vi "Main.vi"(11 "Module Admin":refnum<class "Delacor_lib_QMH_Module Admin.lvclass">) -> ()   [LabVIEW 2024, in "Anode.lvlib"]
doc: "This template is based from the Queued Message Handler design pattern and the Queued Message Handler Project Template that ships with LabVIEW 2014.\n\nThe main difference is that the Queue is private to this module and communication between modules is done via Broadcast and Request events.\n\nRequest events are wrapped via public API methods and are handled in the Event handler loop in this VI.\nAny module can register for Broadcast events sent by this module.\n\nThe Event Handling Loop generates messages based on user interface actions.\n\nThe Message Handling Loop processes messages generated by the Event Handling Loop, or by other messages. The messages are string values, so new messages can be added easily to the Message Cases case structure in the Message Handling Loop. Each message cluster can also provide an optional value for Message Data, which is a variant that can be converted to whatever message-specific data is required.\n_____\nBased on Delacor QMH Project Template 3.1.0.34.\n\n<b>Note:</b> This VI was modified by the <b>Validate DQMH Module</b> tool to add a call to the Error Reported VI at the end of the 'Exit' MHL frame.\n\n<b>Note:</b> This VI was modified by the <b>Validate DQMH Module</b> tool to call the Release Message Queue VI in the top-level Error case.\n\n<b>Note:</b> This VI was modified by the <b>Validate DQMH Module</b> tool to wrap the FP.Open method in the module close code with a Conditional Disable Structure so it does not execute when the Main VI is running as a built EXE."
uses:
  Anode.lvlib
  <vilib>/Delacor/Delacor QMH/Libraries/Module Admin_class/Delacor_lib_QMH_Module Admin.lvclass
  <vilib>/MGI/Panel Manager/Panel/Panel/Panel.lvclass
  Modbus Flexi-Flow API/Fmeasure (F,P1,P2)--cluster.ctl
  Module Data--cluster.ctl
  <vilib>/Plasmionique/MB Master/MB_Master_TCP/MB_Master_TCP.lvclass
  C:/Program Files/National Instruments/LabVIEW 2025/vi.lib/Plasmionique/MB Master/MB_Master/MB_Master.lvclass
  Anode Solenoid Valve--enum.ctl
  Modbus Config--cluster.ctl
  Purge Strategy--cluster.ctl
  Purge Strategy--enum.ctl
  <vilib>/Utility/miscctls.llb/LVPointTypeDef.ctl
  phlair-busch-can-bus/PumpControls.ctl
  phlair-busch-can-bus/CAN Frame Sessions.ctl
  Initialise Pressure Regulator Interface Argument--cluster.ctl
  <vilib>/Delacor/Delacor QMH/Libraries/Message Queue_class/Delacor_lib_QMH_Message Queue.lvclass/Delacor_lib_QMH_Message Queue.ctl
  Read Pressure Regulator Status Argument--cluster.ctl
  Stop Argument--cluster.ctl
  <vilib>/Delacor/Delacor QMH/Libraries/Module Admin_class/Delacor_lib_QMH_Module Admin.lvclass/Delacor_lib_QMH_Module Admin.ctl
  Set Anode Inlet Pressure SP Argument--cluster.ctl
  Set Pressure Regulator Control Function Argument--cluster.ctl
  Modbus Flexi-Flow API/Control Function Values--enum.ctl
  Set Anode Inlet Flow SP Argument--cluster.ctl
  Set Anode Inlet Valve State Argument--cluster.ctl
  Set Anode Gas Supply Valve Argument--cluster.ctl
  Set Purge Valve Argument--cluster.ctl
  Set Purge Strategy Argument--cluster.ctl
  Wake Purge Helper Loop Argument--cluster.ctl
  Reset Counter Argument--cluster.ctl
  Start H2 Sensor Measurement Argument--cluster.ctl
  Stop H2 Sensor Measurement Argument--cluster.ctl
  Modbus Flexi-Flow API/Valve State--enum.ctl
  <vilib>/DAQmx/write.llb/DAQmx Write (Digital Bool 1Line 1Point).vi
  <vilib>/Delacor/Delacor QMH/Libraries/Message Queue_class/Delacor_lib_QMH_Enqueue Message (Single).vi
  <vilib>/Delacor/Delacor QMH/Libraries/Module Admin_class/Delacor_lib_QMH_Get External Launch.vi
  <vilib>/MGI/Panel Manager/Panel/Panel/Window/Window.lvclass
  C:/Program Files/National Instruments/LabVIEW 2025/vi.lib/MGI/Panel Manager/Panel/Panel/Panel.lvclass
  <vilib>/MGI/Panel Manager/Panel/Panel/Window/Window.vi
  <vilib>/DAQmx/miscellaneous.llb/DAQmx Fill In Error Info.vi
  <vilib>/Utility/error.llb/Error Cluster From Error Code.vi
  <vilib>/ErrorRing/Error Ring.xnode
  <vilib>/Delacor/Delacor QMH/Libraries/Message Queue_class/Delacor_lib_QMH_Message Queue.lvclass
  <vilib>/MGI/Panel Manager/Panel/Panel Helper/Panel Helper.lvclass
  Modbus Flexi-Flow API/Bronkhorst Flexi-Flow ModbusTCP API.lvlib
  <vilib>/MGI/Panel Manager/Panel/Panel.lvlib
  phlair-busch-can-bus/phlair-busch-can-bus.lvlib
  <userlib>/_OpenG.lib/error/error.llb/openg_error.lvlib
  <resource>/objmgr/xnet.rc
panel:
  out "H2 Sensor Data":dbl[](array[numeric]) caption="data" format="%.2f"
  out "Counter In":sgl
  out "Data Cluster":T1={"Status"="Initial Message", "MB_TCP session"=refnum, "Flow Rate SP (Valve Shutoff)"=0.0, "Anode Solenoid Valve"=enum."CLOSED", "Fmeasure (F, P1, P2)"={"Fmeasure (F)"=0.0, "Fmeasure (P1)"=0.0, "Fmeasure (P2)"=0.0}, "Anode Status Map"={}, "Modbus Config"={"IP Address"="localhost", "Port (502)"=502, "Slave ID (255)"=255, "Timeout (10000)"=10000}, "DAQmx Task Gas Supply"="", "DAQmx Task Purge Valve"="V203_Anode_Purge_Valve", "Purge Strategy"={"Strategy"=enum."FORCE OFF", "Purge Interval [s]"=30.0, "Purge Duration [s]"=1.0}}
  out "Value":sgl
  out "P2 Setpoint":sgl
  out "Control Function":u16
  out "Fmeasure (F, P1, P2)":T3
  in  "Panel":refnum<class "Panel.lvclass">
  in  "Simulate MHL Error":bool
  in  "Simulate EHL Error":bool
  out "error out":errorcluster
  out "Status":string="Anode Tester sent Stop Message."
  # "This is a template that creates a DQMH Singleton using the MGI Panel Manager Framwork.\n\nImplement your user interface on this front panel. The Panel Manager Framework will manage showing and hiding the panel in the appropriate spot. \n\nSee the block diagram for more information on how to use this template."
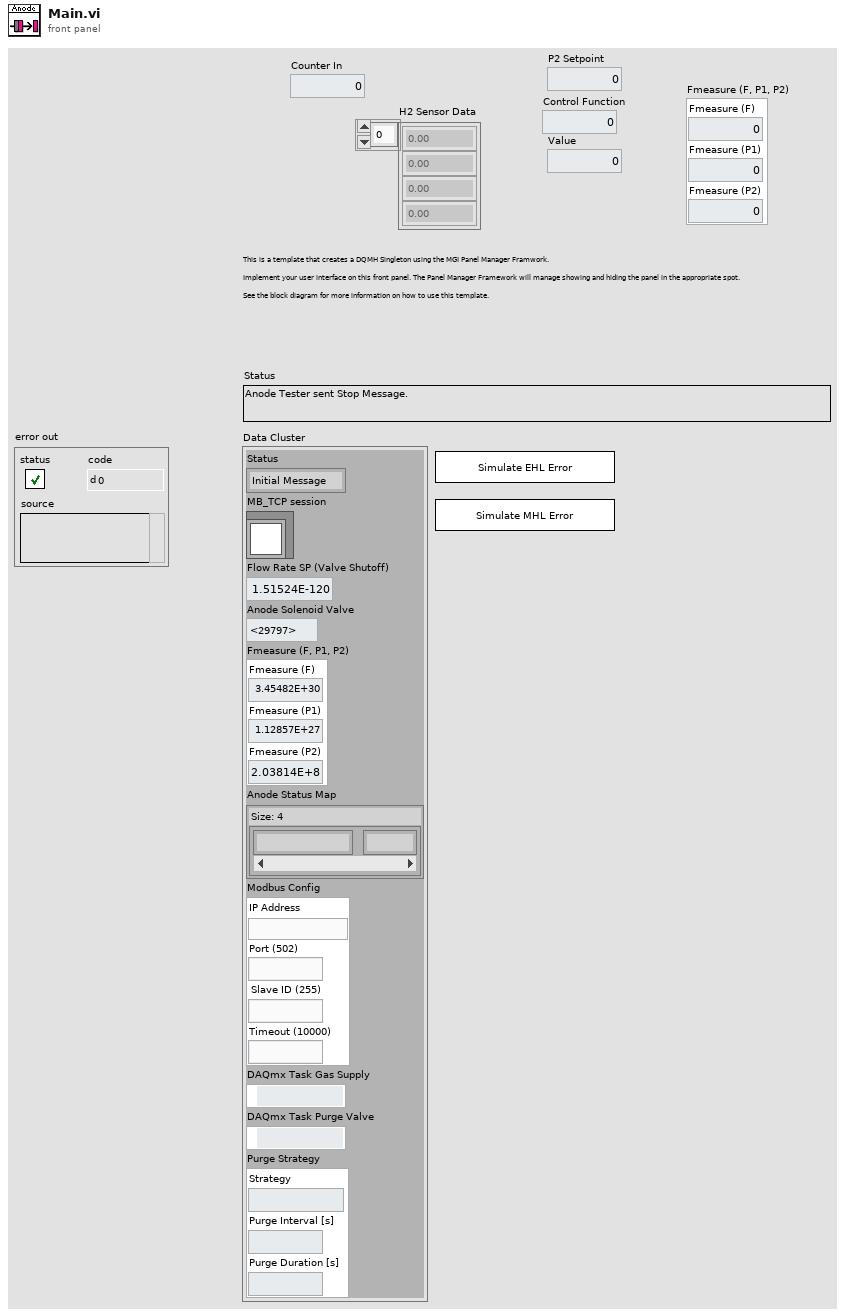
[diagram p1: front panel]
types:
  T1 = typedef "Anode.lvlib/Module Data--cluster.ctl" = cluster{"Status":string, "MB_TCP session":refnum<class "MB_Master_TCP.lvclass">, "Flow Rate SP (Valve Shutoff)":dbl, "Anode Solenoid Valve":T2, "Fmeasure (F, P1, P2)":T3, "Anode Status Map":map{string, dbl}, "Modbus Config":T4, "DAQmx Task Gas Supply":refnum<k21>, "DAQmx Task Purge Valve":refnum<k21>, "Purge Strategy":T5}
  T2 = typedef "Anode.lvlib/Anode Solenoid Valve--enum.ctl" = enum16{"CLOSED", "OPEN"}
  T3 = typedef "Bronkhorst Flexi-Flow ModbusTCP API.lvlib/Fmeasure (F,P1,P2)--cluster.ctl" = cluster{"Fmeasure (F)":sgl, "Fmeasure (P1)":sgl, "Fmeasure (P2)":sgl}
  T4 = typedef "Anode.lvlib/Modbus Config--cluster.ctl" = cluster{"IP Address":string, "Port (502)":u16, "Slave ID (255)":u8, "Timeout (10000)":i32}
  T5 = typedef "Anode.lvlib/Purge Strategy--cluster.ctl" = cluster{"Strategy":T6, "Purge Interval [s]":dbl, "Purge Duration [s]":dbl}
  T6 = typedef "Anode.lvlib/Purge Strategy--enum.ctl" = enum16{"FORCE OFF", "FORCE ON", "TIMED"}
  T7 = typedef "LVPointTypeDef.ctl" = cluster{"Horizontal":i16, "Vertical":i16}
  T8 = typedef "Anode.lvlib/Request Events--cluster.ctl" = cluster{"Stop Module":refnum<user-event>, "Show Panel":refnum<user-event>, "Hide Panel":refnum<user-event>, "Get Module Execution Status":refnum<user-event>, "Show Diagram":refnum<user-event>, "Change Panel":refnum<user-event>, "Set Anode Inlet Pressure SP":refnum<user-event>, "Initialise Pressure Regulator Interface":refnum<user-event>, "Start Polling Pressure Regulator Status":refnum<user-event>, "Stop Polling Pressure Regulator Status":refnum<user-event>, "Read Pressure Regulator Status":refnum<user-event>, "Set Pressure Regulator Control Function":refnum<user-event>, "Set Anode Inlet Flow SP":refnum<user-event>, "Set Anode Inlet Valve State":refnum<user-event>, "Private":cluster{"Wake Connection Helper Loop":refnum<user-event>}, "Set Anode Gas Supply Valve":refnum<user-event>, "Set Purge Valve":refnum<user-event>, "Set Purge Strategy":refnum<user-event>, "Private.Wake Purge Strategy Helper Loop":refnum<user-event>, "Private.Update Purge Strategy Settings":refnum<user-event>, "Wake Purge Helper Loop":refnum<user-event>, "Wake Recirculation Pump Helper Loop":refnum<user-event>, "Sleep Recirculation Pump Helper Loop":refnum<user-event>, "Set Pump Speed SP":refnum<user-event>, "Set Pump Enable State":refnum<user-event>, "Set Pump Speed Control Mode":refnum<user-event>, "Private.Update Purge Strategy Helper Loop":refnum<user-event>, "Force Purge":refnum<user-event>, "Reset Counter":refnum<user-event>, "Private.Wake H2 Sensor Loop":refnum<user-event>, "Private.Sleep H2 Sensor Loop":refnum<user-event>, "Start H2 Sensor Measurement":refnum<user-event>, "Stop H2 Sensor Measurement":refnum<user-event>}
  T9 = typedef "Panel.lvlib/Panel Helper.lvclass/Panel Events.ctl" = cluster{"My Panel":refnum<user-event>, "Top Level Initialized":refnum<user-event>}
  T10 = typedef "phlair-busch-can-bus.lvlib/PumpControls.ctl" = cluster{"Enable Pump":enum16{"DISABLE", "ENABLE"}, "Mass Flow SP [kg/h]":dbl, "Speed SP [U/ min]":u16, "Pump Speed Control":enum16{"DISABLE", "ENABLE"}, "Enable Mass Flow Governer":enum8{"Disable", "Enable", "", "NA"}}
  T11 = typedef "phlair-busch-can-bus.lvlib/CAN Frame Sessions.ctl" = cluster{"Session_Control":refnum<k21>, "Session_Params":refnum<k21>, "Session_Actuals":refnum<k21>, "Session_Acknowledge":refnum<k21>, "Session_H2_Sensor":refnum<k21>}
  T12 = typedef "Anode.lvlib/Initialise Pressure Regulator Interface Argument--cluster.ctl" = cluster{"Modbus Config":T4}
  T13 = typedef "Anode.lvlib/Read Pressure Regulator Status Argument--cluster.ctl" = cluster{"Boolean":bool}
  T14 = typedef "Anode.lvlib/Stop Argument--cluster.ctl" = cluster{"Origin":string, "Exit via Stop Module Req?":bool, "Wait for Module to stop?":bool}
  T15 = typedef "Anode.lvlib/Set Anode Inlet Pressure SP Argument--cluster.ctl" = cluster{"Anode Inlet Pressure [bar]":dbl}
  T16 = typedef "Anode.lvlib/Set Pressure Regulator Control Function Argument--cluster.ctl" = cluster{"Function":T17}
  T17 = typedef "Bronkhorst Flexi-Flow ModbusTCP API.lvlib/Control Function Values--enum.ctl" = enum16{"Flow", "Upstream pressure", "Downstream pressure", "Flow with upstream pressure limit", "Flow with downstream pressure limit", "Upstream pressure with flow limit", "Downstream pressure with flow limit"}
  T18 = typedef "Anode.lvlib/Set Anode Inlet Flow SP Argument--cluster.ctl" = cluster{"Flow SP [slm]":dbl}
  T19 = typedef "Anode.lvlib/Set Anode Inlet Valve State Argument--cluster.ctl" = cluster{"Anode Solenoid Valve":T2}
  T20 = typedef "Anode.lvlib/Set Anode Gas Supply Valve Argument--cluster.ctl" = cluster{"Valve State":enum16{"CLOSED", "OPEN"}}
  T21 = typedef "Anode.lvlib/Set Purge Valve Argument--cluster.ctl" = cluster{"Valve State":enum16{"CLOSED", "OPEN"}}
  T22 = typedef "Anode.lvlib/Set Purge Strategy Argument--cluster.ctl" = cluster{"Purge Controller":T5}
  T23 = typedef "Anode.lvlib/Wake Purge Helper Loop Argument--cluster.ctl" = cluster{"Boolean":bool}
  T24 = typedef "Anode.lvlib/Reset Counter Argument--cluster.ctl" = cluster{"Boolean":bool}
  T25 = typedef "Anode.lvlib/Start H2 Sensor Measurement Argument--cluster.ctl" = cluster{"Boolean":bool}
  T26 = typedef "Anode.lvlib/Stop H2 Sensor Measurement Argument--cluster.ctl" = cluster{"Boolean":bool}
  T27 = enum32{"invalid lock state", "Not Locked", "Locked (No Password)", "Password-protected"}
  T28 = typedef "Bronkhorst Flexi-Flow ModbusTCP API.lvlib/Valve State--enum.ctl" = enum16{"Close", "Open"}
  T29 = enum16{"No reset", "Reset counter", "Reset alarm", "Reset counter (all)", "Reset and disable counter", "Reset firmware program (soft reset)", "Reset Alarm infor error bit", "Reset Alarm info warning bit"}
  T30 = typedef "Anode.lvlib/Purge Valve State--cluster.ctl" = enum16{"WAITING", "PURGING"}
  T31 = cluster{"Timestamp Latest Purge":timestamp, "Timestamp Purge Start":timestamp, "Purge State":T30}
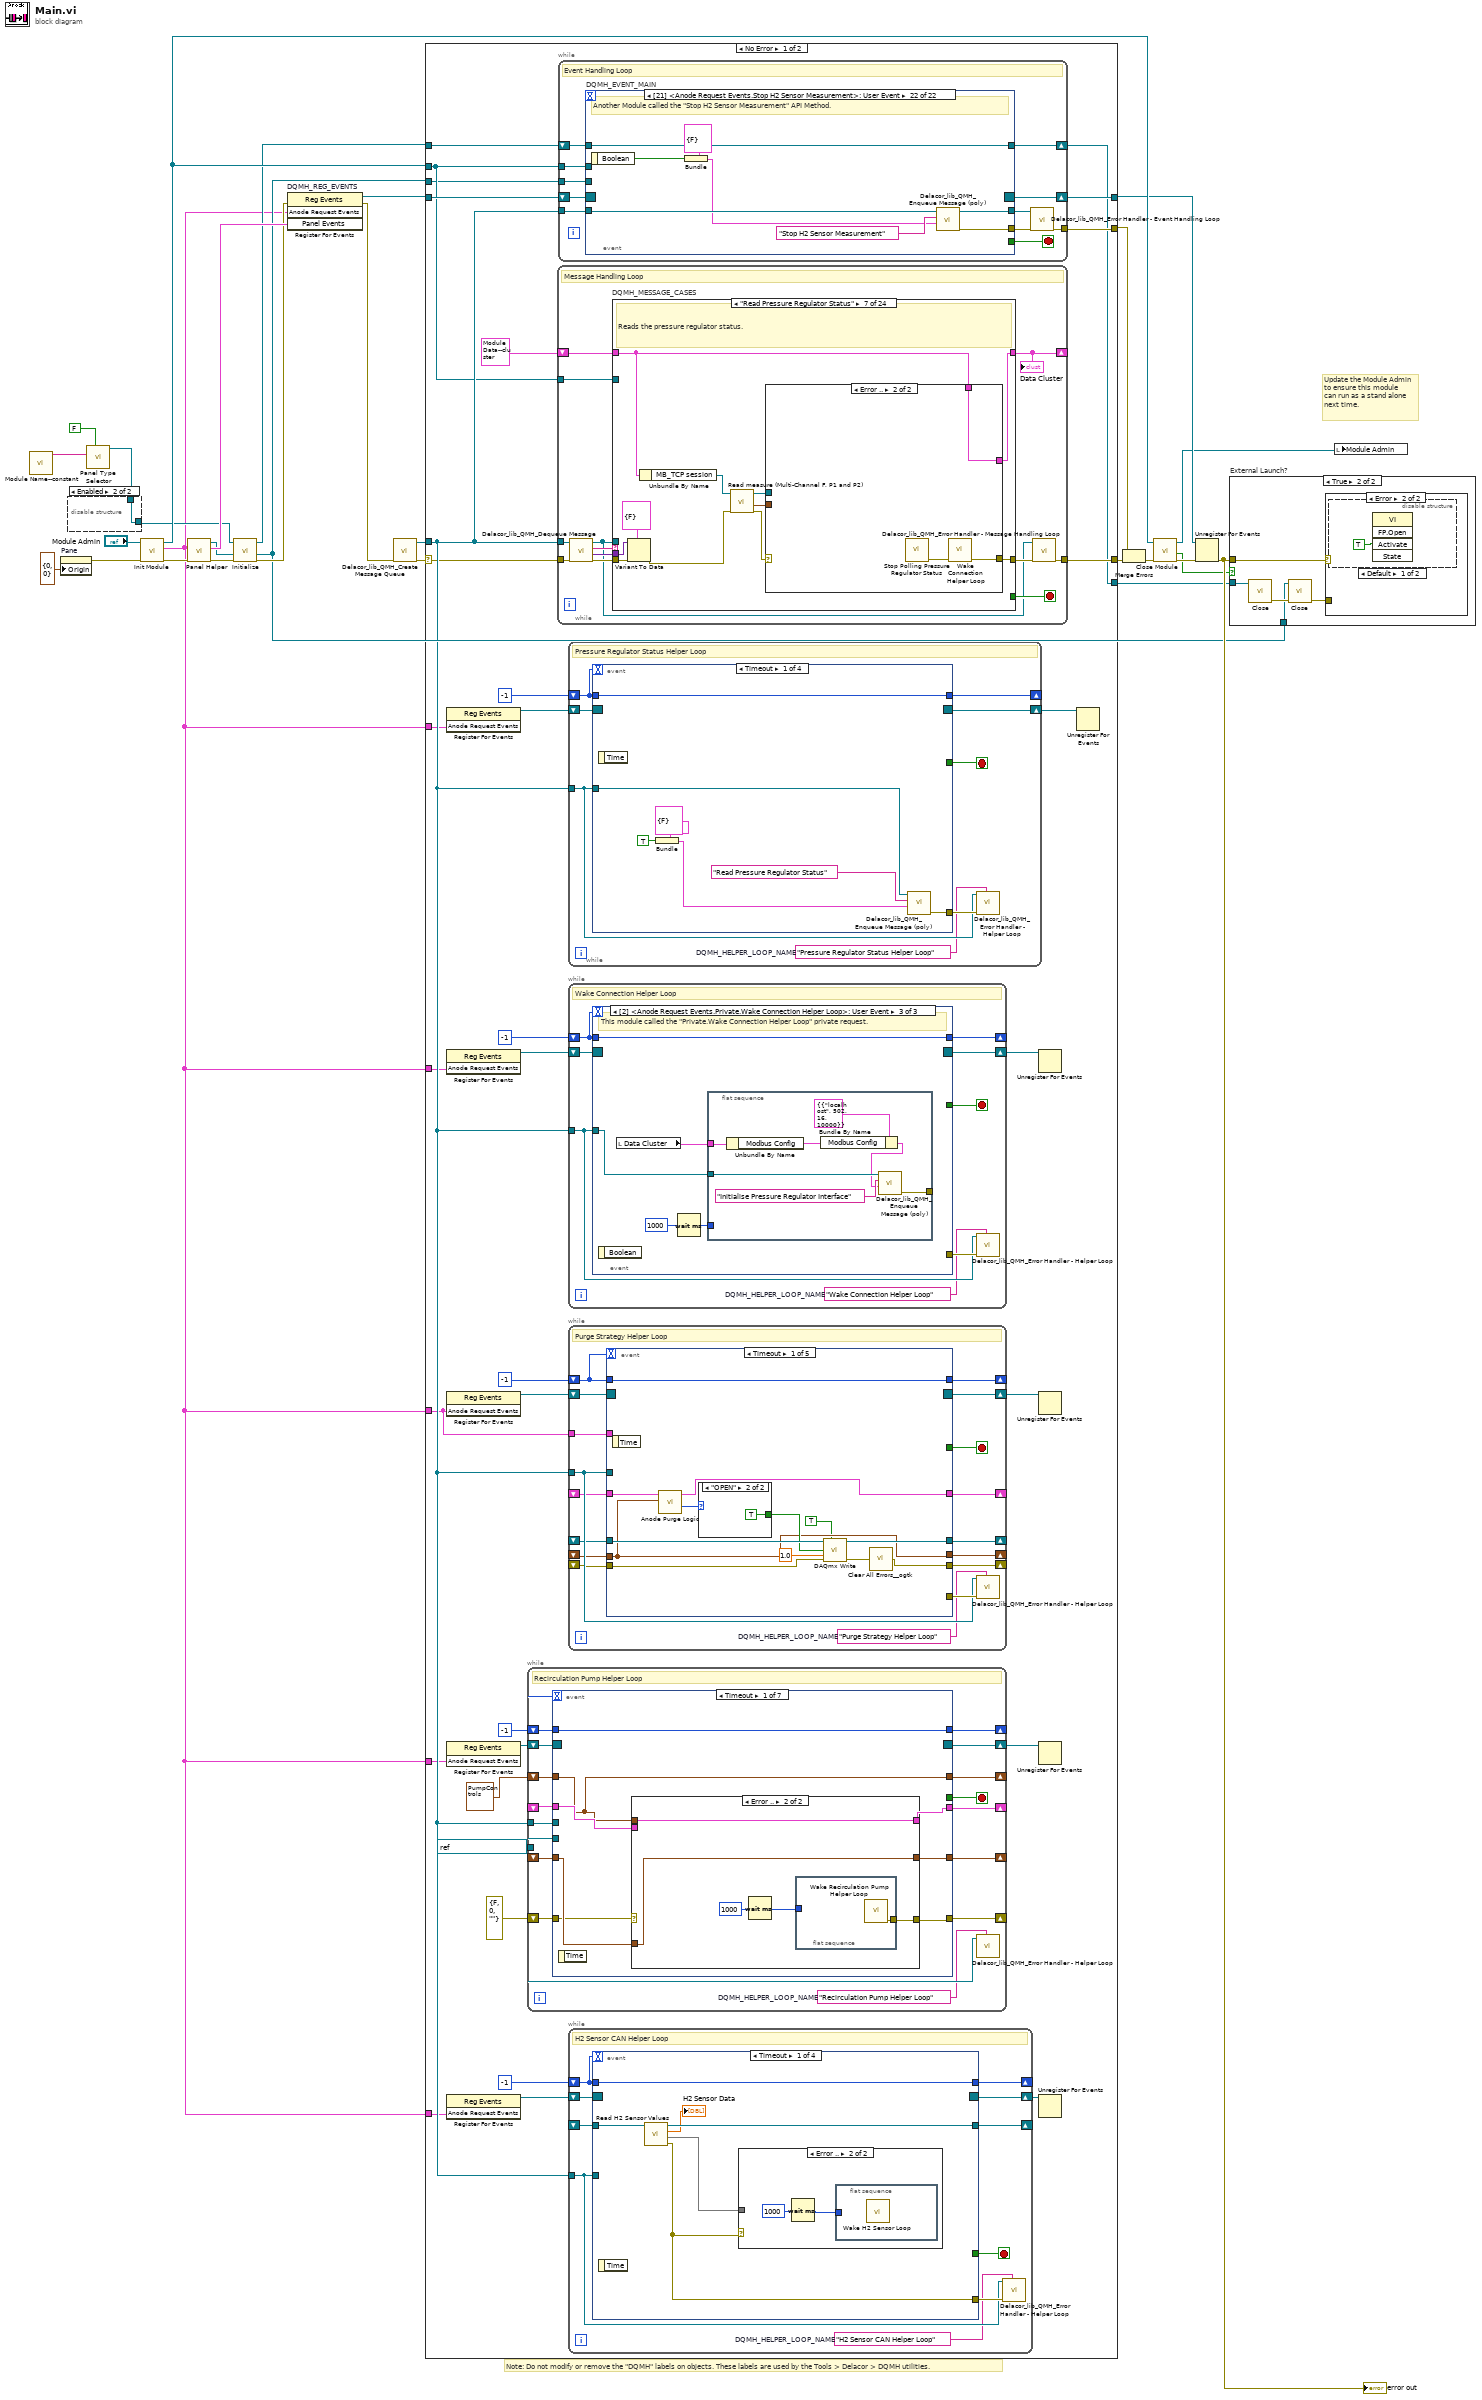
[diagram p0: block diagram]
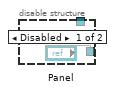
[diagram p2: hidden frame]
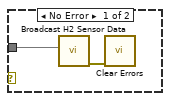
[diagram p6: hidden frame]
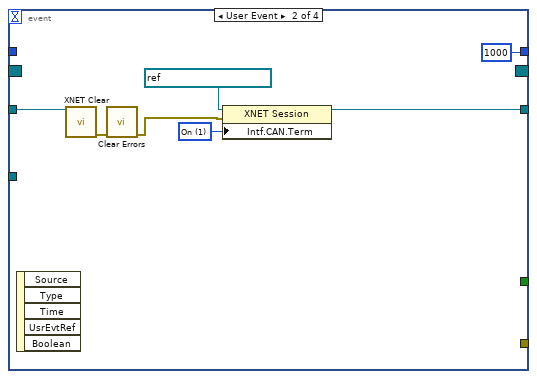
[diagram p7: hidden frame]
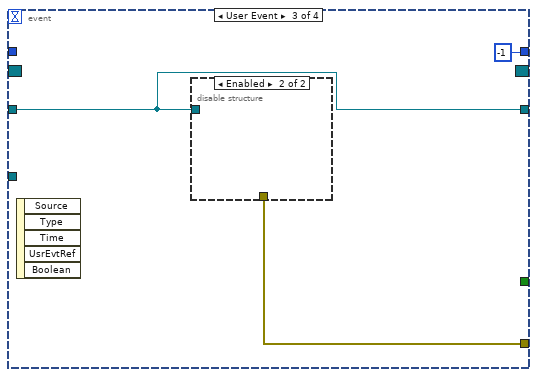
[diagram p8: hidden frame]
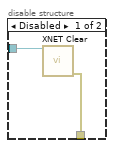
[diagram p9: hidden frame]
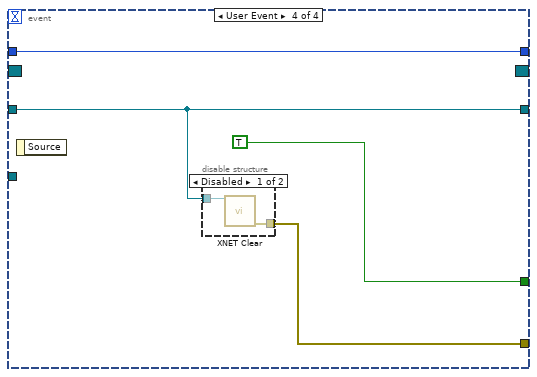
[diagram p10: hidden frame]
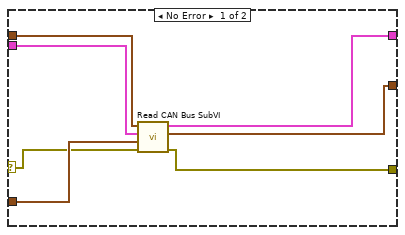
[diagram p12: hidden frame]
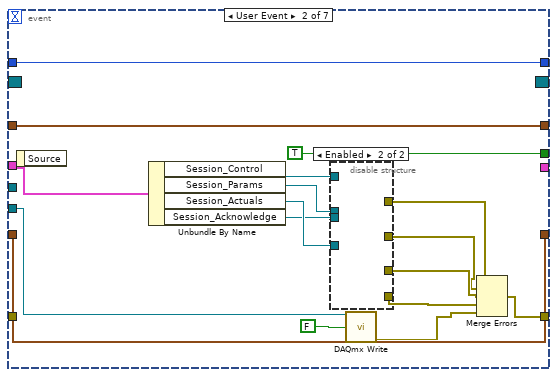
[diagram p13: hidden frame]
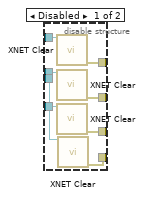
[diagram p14: hidden frame]
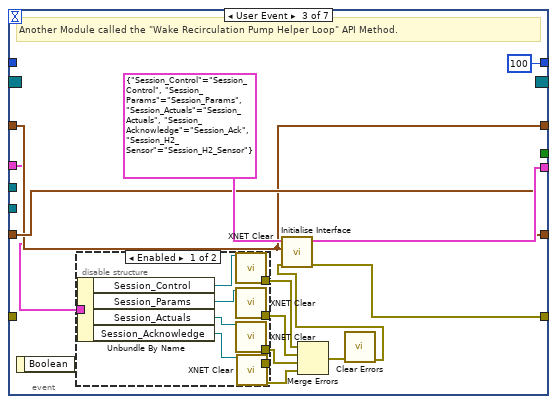
[diagram p15: hidden frame]
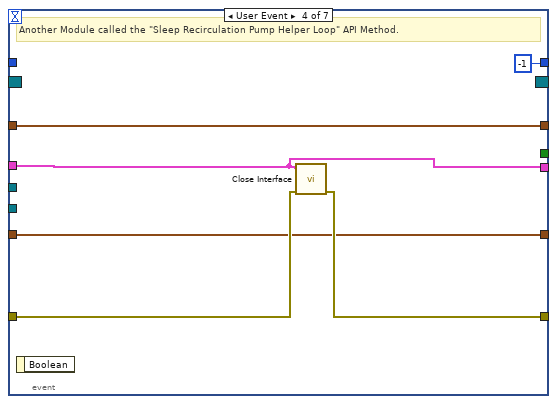
[diagram p17: hidden frame]
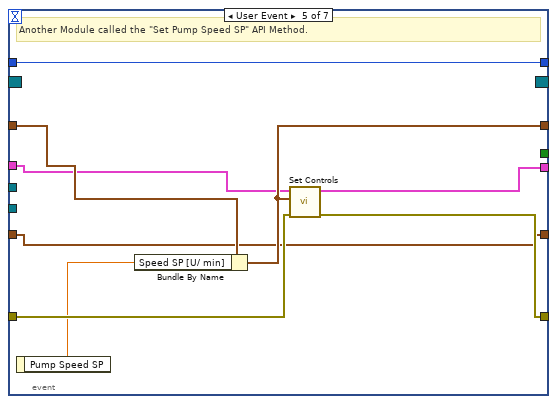
[diagram p18: hidden frame]
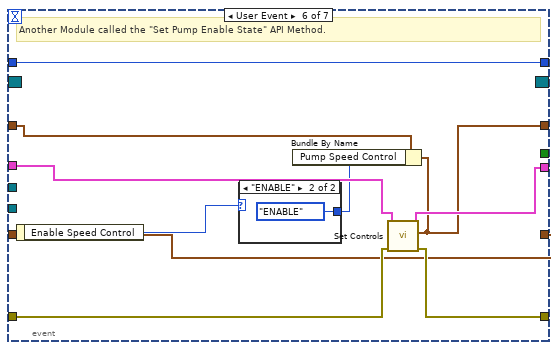
[diagram p19: hidden frame]
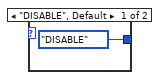
[diagram p20: hidden frame]
diagram:
  # "Note: Do not modify or remove the \"DQMH\" labels on objects. These labels are used by the Tools > Delacor > DQMH utilities."
  # "Update the Module Admin to ensure this module can run as a stand alone next time."
  n1 = call "Module Name--constant.vi"() -> ("Module Name"=w2:string)  [unwired: 11 in]
  n2 = property on="Pane" class="Pane"("Origin"=T7 {"Horizontal"=0, "Vertical"=0}) -> (error out=w5:errorcluster)  [unwired: 2 in, 1 out]
  n3 = call-poly <vilib>:"Panel Type Selector.vi"("Autoshow? (T)"=FALSE, "Default Title"=w2) -> ("Window out"=w3:refnum<class "Window.lvclass">)  [unwired: 8 in, 1 out]
  n4 = disable-structure shown="Enabled" {
    disable-tunnel: ["Panel" w31] -> w10
    disable-tunnel: w3 -> [_ w31]
    frame Disabled {
    }
    frame Enabled {
    }
  }
  n5 = call "Init Module.vi"("error in (no error)"=w5, "Singleton Module Admin in"="Module Admin") -> ("error out"=w15:errorcluster, "Anode Request Events"=w1:T8, "Singleton Module Admin out"=w29:refnum<class "Delacor_lib_QMH_Module Admin.lvclass">)  [unwired: 7 in]
  n6 = call <vilib>:"Panel Helper.vi"("Error In"=w15) -> ("Error Out"=w12:errorcluster, "Panel Events"=w14:T9, "Panel Helper out"=w11:refnum<class "Panel Helper.lvclass">)  [unwired: 8 in]
  n7 = call <vilib>:"Initialize.vi"("error in (no error)"=w12, "My Helper in"=w11, "Panel In"=w10) -> ("error out"=w9:errorcluster, "My Helper out"=w8:refnum<class "Panel Helper.lvclass">, "Panel Out"=w7:refnum<class "Window.lvclass">)  [unwired: 6 in]
  n8 = register-events "DQMH_REG_EVENTS"(error in=w9, w1, w14) -> (reference out=w26:refnum<event-registration>, error out=w13:errorcluster)  [unwired: 1 in]
  n9 = call <vilib>:"Delacor_lib_QMH_Create Message Queue.vi"("error in"=w13) -> ("error out"=w17:errorcluster, "Message Queue"=w25:refnum<class "Delacor_lib_QMH_Message Queue.lvclass">)  [unwired: 9 in]
  n10 = case shown="No Error" w17 {
    selector: w17 -> [w59 w823]
    tunnel: [w65 w823] -> w28
    tunnel: [w64 w828] -> w27
    tunnel: w26 -> [w62 w828]
    tunnel: w25 -> [w61 w819]
    tunnel: [w60 _] -> w21
    tunnel: w29 -> [w58 w824]
    tunnel: w7 -> [w56 w820]
    tunnel: w8 -> [w57 _]
    tunnel: [w55 w820] -> w16
    tunnel: w1 -> [w54 _]
    tunnel: w1 -> [w50 _]
    tunnel: w1 -> [w38 _]
    tunnel: w1 -> [w43 _]
    tunnel: w1 -> [w36 _]
    frame No Error {
      n11 = register-events ("DQMH_HELPER_REGFOREVENTS")(w54) -> (reference out=w52:refnum<event-registration>)  [unwired: 2 in, 1 out]
      n12 = register-events ("DQMH_HELPER_REGFOREVENTS")(w50) -> (reference out=w48:refnum<event-registration>)  [unwired: 2 in, 1 out]
      n13 = register-events ("DQMH_HELPER_REGFOREVENTS")(w38) -> (reference out=w45:refnum<event-registration>)  [unwired: 2 in, 1 out]
      n14 = register-events ("DQMH_HELPER_REGFOREVENTS")(w43) -> (reference out=w41:refnum<event-registration>)  [unwired: 2 in, 1 out]
      n15 = register-events ("DQMH_HELPER_REGFOREVENTS")(w36) -> (reference out=w34:refnum<event-registration>)  [unwired: 2 in, 1 out]
      n16 = while "DQMH_HELPER_LOOP" {
        shift-right: [w119] -> _
        shift-left: -1 -> [w118]
        shift-right: [w116] -> w42
        shift-left: w41 -> [w117]
        tunnel: w61 -> [w114]
        shift-right: [w111] -> _
        shift-left: _ -> [w112]
        shift-right: [w109] -> _
        shift-left: errorcluster {"status"=FALSE, "code"=0, "source"=""} ("error out") -> [w110]
        shift-right: [w108] -> _
        shift-left: T10 {"Enable Pump"=enum."DISABLE", "Mass Flow SP [kg/h]"=0.0, "Speed SP [U/ min]"=0, "Pump Speed Control"=enum."DISABLE", "Enable Mass Flow Governer"=enum."Disable"} ("Initial Pump Controls") -> [w107]
        shift-right: [w106] -> _
        shift-left: _ -> [w105]
        tunnel: refnum<k21> "H2_Pump_On" ("task/channels in") -> [w104]
        stop <- w115 stop-if-true
        w113 = "Recirculation Pump Helper Loop"  # DQMH_HELPER_LOOP_NAME
        # "Recirculation Pump Helper Loop"
        n17 = event "DQMH_HELPER_EVENT_STRUCTURE" shown="[0] Timeout" {
          selector: w117 -> [_ _ _ _ _ _ _]
          dyn-events: [_ _ _ _ _ _ _] -> w116
          timeout: w118 -> [_ _ _ _ _ _ _]
          tunnel: w118 -> [w127 w157 _ _ w194 w203 w217]
          tunnel: [w127 w157 100 ("Timeout (s)") -1 ("Timeout (s)") w194 w203 w216] -> w119
          tunnel: [_ TRUE _ _ _ _ _] -> w115
          tunnel: w114 -> [_ _ _ _ _ _ _]
          tunnel: w112 -> [w124 w151 w172 w191 w197 w209 _]
          tunnel: [w125 _ w177 w191 w196 w208 _] -> w111
          tunnel: w110 -> [w120 _ _ w190 w202 w212 _]
          tunnel: [w126 w145 w178 w189 w201 w211 w223] -> w109
          tunnel: [w123 w152 w173 w192 w198 w207 w219] -> w108
          tunnel: w107 -> [w123 w152 w173 w192 w199 w210 w220]
          tunnel: [w122 w155 w174 w188 w195 w206 w227] -> w106
          tunnel: w105 -> [w121 w155 w174 w188 w195 w206 w227]
          tunnel: w104 -> [_ w154 _ _ _ _ w215]
          event Timeout {
            n18 = event-data() -> ()  [unwired: 1 in, 1 out]
            n19 = case shown="Error .." w120 {
              selector: w120 -> [w129 _]
              tunnel: [w128 w139] -> w126
              tunnel: [w134 w137] -> w125
              tunnel: w124 -> [w133 w137]
              tunnel: w123 -> [w132 _]
              tunnel: [w131 w138] -> w122
              tunnel: w121 -> [w130 w138]
              frame No Error {
                n20 = call "Read CAN Bus SubVI.vi"("error in (no error)"=w129, "seconds since 1Jan1904 in"=w130, "output cluster in"=w133, "Initial Pump Controls"=w132) -> ("error out"=w128:errorcluster, "seconds since 1Jan1904 out"=w131:timestamp, "output cluster out"=w134:T11)  [unwired: 5 in]
              }
              frame Error {
                n21 = Wait (ms)(milliseconds to wait=u32 1000) -> (millisecond timer value=w135:u32)
                n22 = flat-sequence {
                  tunnel: [w140] -> w139
                  tunnel: w135 -> [_]
                  frame #0 {
                    n23 = call "Wake Recirculation Pump Helper Loop.vi"() -> ("error out"=w140:errorcluster)  [unwired: 11 in]
                  }
                }
              }
            }
          }
          event User Event {
            n24 = event-data() -> ()  [unwired: 1 in, 1 out]
            n25 = Unbundle By Name(w151) -> ("Session_Control"=w150:refnum<k21>, "Session_Params"=w149:refnum<k21>, "Session_Actuals"=w148:refnum<k21>, "Session_Acknowledge"=w147:refnum<k21>)
            n26 = disable-structure shown="Enabled" {
              disable-tunnel: w150 -> [w165 _]
              disable-tunnel: w149 -> [w164 _]
              disable-tunnel: w148 -> [w163 _]
              disable-tunnel: w147 -> [w162 _]
              disable-tunnel: [w161 _] -> w144
              disable-tunnel: [w160 _] -> w143
              disable-tunnel: [w159 _] -> w142
              disable-tunnel: [w158 _] -> w141
              frame Disabled {
                n27 = call <vilib>:"XNET Clear.vi"("session in"=w165) -> ("error out"=w158:errorcluster)  [unwired: 14 in]
                n28 = call <vilib>:"XNET Clear.vi"("session in"=w164) -> ("error out"=w159:errorcluster)  [unwired: 14 in]
                n29 = call <vilib>:"XNET Clear.vi"("session in"=w163) -> ("error out"=w160:errorcluster)  [unwired: 14 in]
                n30 = call <vilib>:"XNET Clear.vi"("session in"=w162) -> ("error out"=w161:errorcluster)  [unwired: 14 in]
              }
              frame Enabled {
              }
            }
            n31 = call-poly <vilib>:"DAQmx Write.vi"("task/channels in"=w154, "data"=FALSE) -> ("error out"=w146:errorcluster)  [unwired: 11 in, 2 out]
            n32 = Merge Errors(w141, w142, w143, w144, w146) -> (w145:errorcluster)
          }
          event User Event {
            # "Another Module called the \"Wake Recirculation Pump Helper Loop\" API Method."
            n33 = event-data() -> ()  [unwired: 1 in, 1 out]
            n34 = disable-structure shown="Enabled" {
              disable-tunnel: w172 -> [w187 _]
              disable-tunnel: [w182 _] -> w171
              disable-tunnel: [w181 _] -> w170
              disable-tunnel: [w180 _] -> w169
              disable-tunnel: [w179 _] -> w168
              frame Enabled {
                n35 = Unbundle By Name(w187) -> ("Session_Control"=w186:refnum<k21>, "Session_Params"=w185:refnum<k21>, "Session_Actuals"=w184:refnum<k21>, "Session_Acknowledge"=w183:refnum<k21>)
                n36 = call <vilib>:"XNET Clear.vi"("session in"=w186) -> ("error out"=w182:errorcluster)  [unwired: 14 in]
                n37 = call <vilib>:"XNET Clear.vi"("session in"=w185) -> ("error out"=w181:errorcluster)  [unwired: 14 in]
                n38 = call <vilib>:"XNET Clear.vi"("session in"=w184) -> ("error out"=w180:errorcluster)  [unwired: 14 in]
                n39 = call <vilib>:"XNET Clear.vi"("session in"=w183) -> ("error out"=w179:errorcluster)  [unwired: 14 in]
              }
              frame Disabled {
              }
            }
            n40 = Merge Errors(w171, w170, w169, w168) -> (w167:errorcluster)
            n41 = call <vilib>:"Clear Errors.vi"("error in (no error)"=w167) -> ("error out"=w166:errorcluster)  [unwired: 5 in, 1 out]
            n42 = call "Initialise Interface.vi"("error in (no error)"=w166, "Initial Pump Controls"=w173, "CAN Frame Sessions"=T11 {"Session_Control"="Session_Control", "Session_Params"="Session_Params", "Session_Actuals"="Session_Actuals", "Session_Acknowledge"="Session_Ack", "Session_H2_Sensor"="Session_H2_Sensor"}) -> ("error out"=w178:errorcluster, "output cluster"=w177:T11)  [unwired: 7 in]
          }
          event User Event {
            # "Another Module called the \"Sleep Recirculation Pump Helper Loop\" API Method."
            n43 = event-data() -> ()  [unwired: 1 in, 1 out]
            n44 = call "Close Interface.vi"("error in (no error)"=w190, "CAN Frame Sessions"=w191) -> ("error out"=w189:errorcluster)  [unwired: 9 in]
          }
          event User Event {
            # "Another Module called the \"Set Pump Speed SP\" API Method."
            n45 = event-data() -> ("Pump Speed SP"=w200:dbl)  [unwired: 1 in]
            n46 = Bundle By Name(cluster=w199, "Speed SP [U/ min]"=w200) -> (w198:T10)
            n47 = call "Set Controls.vi"("error in (no error)"=w202, "Pump Controls"=w198, "input cluster"=w197) -> ("error out"=w201:errorcluster, "output cluster"=w196:T11)  [unwired: 7 in]
          }
          event User Event {
            # "Another Module called the \"Set Pump Enable State\" API Method."
            n48 = event-data() -> ("Enable Speed Control"=w205:enum8{"DISABLE", "ENABLE"})  [unwired: 1 in]
            n49 = case shown="\"ENABLE\"" w205 {
              tunnel: [enum16{"DISABLE", "ENABLE"}."DISABLE" ("Pump Speed Control") enum16{"DISABLE", "ENABLE"}."ENABLE" ("Pump Speed Control")] -> w204
              frame "DISABLE", Default {
              }
              frame "ENABLE" {
              }
            }
            n50 = Bundle By Name(cluster=w210, "Pump Speed Control"=w204) -> (w207:T10)
            n51 = call "Set Controls.vi"("error in (no error)"=w212, "Pump Controls"=w207, "input cluster"=w209) -> ("error out"=w211:errorcluster, "output cluster"=w208:T11)  [unwired: 7 in]
          }
          event User Event {
            n52 = event-data() -> ("Enable Pump"=w226:enum16{"DISABLE", "ENABLE"})  [unwired: 1 in]
            n53 = case shown="\"ENABLE\"" w226 {
              tunnel: [FALSE TRUE] -> w225
              tunnel: [w230 w234] -> w221
              tunnel: [enum16{"DISABLE", "ENABLE"}."DISABLE" ("Enable Pump") enum16{"DISABLE", "ENABLE"}."ENABLE" ("Enable Pump")] -> w218
              tunnel: w217 -> [_ _]
              tunnel: [-1 100] -> w216
              frame "DISABLE", Default {
                n54 = call "Sleep Recirculation Pump Helper Loop.vi"() -> ("error out"=w230:errorcluster)  [unwired: 11 in]
              }
              frame "ENABLE" {
                n55 = call "Wake Recirculation Pump Helper Loop.vi"() -> ("error out"=w234:errorcluster)  [unwired: 11 in]
              }
            }
            n56 = call-poly <vilib>:"DAQmx Write.vi"("task/channels in"=w215, "auto start"=TRUE, "data"=w225, "error in"=w221) -> ("error out"=w224:errorcluster)  [unwired: 9 in, 2 out]
            n57 = Bundle By Name(cluster=w220, "Enable Pump"=w218) -> (w219:T10)
            n58 = call <vilib>:"Clear Errors.vi"("error in (no error)"=w224) -> ("error out"=w223:errorcluster)  [unwired: 5 in, 1 out]
          }
        }
        n59 = call-dynamic "Delacor_lib_QMH_Error Handler - Helper Loop.vi"("Error Debug"=w113, "Message Queue in"=w114) -> ()  [unwired: 8 in, 2 out]
      }
      n60 = while {
        tunnel: w61 -> [w529]
        shift-right: [w535] -> _
        shift-left: T1 {"Status"="", "MB_TCP session"=refnum, "Flow Rate SP (Valve Shutoff)"=0.0, "Anode Solenoid Valve"=enum."CLOSED", "Fmeasure (F, P1, P2)"={"Fmeasure (F)"=0.0, "Fmeasure (P1)"=0.0, "Fmeasure (P2)"=0.0}, "Anode Status Map"={}, "Modbus Config"={"IP Address"="localhost", "Port (502)"=502, "Slave ID (255)"=255, "Timeout (10000)"=10000}, "DAQmx Task Gas Supply"="", "DAQmx Task Purge Valve"="", "Purge Strategy"={"Strategy"=enum."FORCE OFF", "Purge Interval [s]"=30.0, "Purge Duration [s]"=1.0}} ("Data Cluster") -> [w536]
        tunnel: w59 -> [w533]
        tunnel: [w527] -> w65
        tunnel: w58 -> [w526]
        stop <- w534 stop-if-true
        # "Message Handling Loop"
        n61 = call-dynamic "Delacor_lib_QMH_Dequeue Message.vi"("error in"=w533, "Message Queue in"=w529) -> ("error out"=w532:errorcluster, "Message Data"=w530:variant, "Message"=w531:string, "Message Queue out"=w528:refnum<class "Delacor_lib_QMH_Message Queue.lvclass">)  [unwired: 6 in]
        n62 = case "DQMH_MESSAGE_CASES" shown="\"Read Pressure Regulator Status\"" w531 {
          selector: w531 -> [_ _ _ _ _ _ _ _ _ _ _ _ _ _ _ _ _ _ _ _ _ _ _ w808]
          tunnel: w528 -> [_ _ _ _ _ _ _ _ _ _ _ _ _ _ _ _ _ _ _ _ w766 w781 w804 _]
          tunnel: w532 -> [w541 w558 w562 w580 w597 w614 w625 w652 w664 w677 w692 w705 w716 w722 w732 w738 w744 w747 w750 w755 w772 w785 w806 _]
          tunnel: [w544 w559 w561 w578 w586 w603 w618 w647 w659 w670 w687 w698 w709 w717 w728 w733 w739 w745 w748 w753 w763 w783 w801 w809] -> w537
          tunnel: w536 -> [w549 w560 w563 w579 w583 w610 w620 w644 w656 w673 w685 w700 w712 w721 w725 w737 w743 w746 w749 w754 w771 w784 w793 w810]
          tunnel: [w548 w560 w563 w579 w588 w609 w619 w643 w655 w672 w684 w700 w711 w721 w724 w737 w743 w746 w749 w754 w771 w784 w793 w810] -> w535
          tunnel: [_ _ _ _ _ _ _ _ _ _ _ _ _ _ _ _ _ _ _ _ _ _ w803 _] -> w534
          tunnel: w530 -> [_ w557 _ _ w596 w613 w624 w651 w663 w676 w691 w704 w715 w720 w731 w736 w742 _ _ _ w770 _ w800 _]
          tunnel: w526 -> [w543 _ _ _ _ _ _ _ _ _ _ _ _ _ _ _ _ _ _ _ w765 _ w795 _]
          frame "Initialize" {
            w547 = "Initial Message" ("Initial Message")
            # "Initialize - Any operation that needs to be done before the module can receive messages. Synchronize Caller Events.vi will inform Start Module.vi that the module has launched and is ready to receive messages. Module Did Init.vi will broadcast that the module initialized."
            n63 = disable-structure shown="Enabled" {
              disable-tunnel: w541 -> [w551 w552]
              disable-tunnel: [w550 w552] -> w540
              frame Disabled {
                n64 = call "Wake Recirculation Pump Helper Loop.vi"("error in"=w551) -> ("error out"=w550:errorcluster)  [unwired: 10 in]
              }
              frame Enabled {
              }
            }
            n65 = call "Synchronize Caller Events.vi"("error in (no error)"=w540, "Singleton Module Admin in"=w543) -> ("error out"=w539:errorcluster)  [unwired: 8 in, 1 out]
            n66 = Bundle By Name(cluster=w549, "Status"=w547, "DAQmx Task Purge Valve"=refnum<k21> "V203_Anode_Purge_Valve") -> (w548:T1)
            n67 = call "Wake Purge Strategy Helper Loop.vi"("error in"=w539) -> ("error out"=w538:errorcluster)  [unwired: 10 in]
            n68 = local write "Status"(w547) -> ()
            n69 = call "Module Name--constant.vi"() -> ("Module Name"=w545:string)  [unwired: 11 in]
            n70 = call "Module Did Init.vi"("error in (no error)"=w538, "Initialized?"=TRUE, "Origin"=w545) -> ("error out"=w544:errorcluster)  [unwired: 8 in]
          }
          frame "Update Display" {
            # "Broadcast updated status to any VI registered to listen to this module's broadcast events."
            # "Convert the message data to a string to display in the Status indicator."
            # "#CodeRecommended - If you wish to decouple the Message Handling Loop from your user interface, consider creating User Events (like the \"Stop\" event in this VI) to message the Event Handling Loop whenever the user interface needs updating."
            # "Update Display - Update user interface here."
            n71 = Variant To Data(error in=w558, type="" ("Empty String Constant"), Variant=w557) -> (data=w555:string, error out=w554:errorcluster)
            "Status" <- w555
            n72 = call "Status Updated.vi"("error in (no error)"=w554, "Status"=w555) -> ("error out"=w553:errorcluster)  [unwired: 9 in]
            n73 = Merge Errors(w553) -> (w559:errorcluster)
          }
          frame "Show Diagram" {
            # "Show Diagram - Show the block diagram of this VI. Used as a debugging tool. There is a button in the module tester that fires the Show Diagram request, which runs this message. Note that the diagram will not be displayed if it is password-protected and the password is not in the cache."
            n74 = disable-structure shown="RUN_TIME_ENGINE==False" {
              disable-tunnel: [w571 w577] -> w561
              disable-tunnel: w562 -> [w570 w577]
              frame condition #0 (active) {
                # "functionality not available in exe"
                n75 = invoke on="Invoke Node" class="VI" method="Lock State.Get"(error in=w570) -> (error out=w569:errorcluster, "Get Lock State"=w568:T27, "pwd in cache"=w565:bool)  [unwired: 3 in, 1 out]
                n76 = Equal?(x=T27."Password-protected", y=w568) -> (x = y?=w566:bool)
                n77 = Compound Arithmetic op=AND(w566, invert w565) -> (w564:bool)
                n78 = case shown="False" w564 {
                  tunnel: [w574 w576] -> w571
                  tunnel: w569 -> [w572 w576]
                  frame False {
                    n79 = property on="Property Node" class="VI"(error in=w572, "BDWin.Open"=TRUE ("Block Diagram Window:Open")) -> (error out=w574:errorcluster)  [unwired: 1 in, 1 out]
                    n80 = call "Status Updated.vi"("Status"="Block Diagram shown." ("format string")) -> ()  [unwired: 10 in, 1 out]
                  }
                  frame True {
                    # "Password-protected VI, and the password is not in the cache. Do not show the diagram."
                  }
                }
              }
              frame condition #1 {
              }
            }
          }
          frame "--- Module Specific ---" {
            # "Separator -- The following cases handle messages specific to this Module."
            n81 = Merge Errors(w580) -> (w578:errorcluster)
          }
          frame "Initialise Pressure Regulator Interface" {
            # "Initialises the pressure regulator interface."
            n82 = Variant To Data(error in=w597, type=T12 {"Modbus Config"={"IP Address"="localhost", "Port (502)"=502, "Slave ID (255)"=16, "Timeout (10000)"=10000}} ("Initialise Pressure Regulator Interface Argument"), Variant=w596) -> (data=w585:T12, error out=w590:errorcluster)
            n83 = Unbundle By Name(w583) -> ("MB_TCP session"=w582:refnum<class "MB_Master_TCP.lvclass">)
            n84 = Unbundle By Name(w585) -> ("Modbus Config"=w584:T4)
            n85 = Unbundle By Name(w585) -> ("Modbus Config.Slave ID (255)"=w594:u8, "Modbus Config.IP Address"=w593:string, "Modbus Config.Port (502)"=w592:u16, "Modbus Config.Timeout (10000)"=w591:i32)
            n86 = call "Modbus TCP Close.vi"("MB session in"=w582) -> ("error out"=w581:errorcluster)  [unwired: 10 in]
            n87 = call <vilib>:"Clear Errors.vi"("error in (no error)"=w581) -> ()  [unwired: 5 in, 2 out]
            n88 = call "Modbus TCP Initialise.vi"("Slave ID (255)"=w594, "error in (no error)"=w590, "Timeout (10000)"=w591, "Port (502)"=w592, "IP Address"=w593) -> ("error out"=w587:errorcluster, "MB_TCP session"=w589:refnum<class "MB_Master_TCP.lvclass">)  [unwired: 5 in]
            n89 = case shown="No Error" w587 {
              selector: w587 -> [w598 w602]
              tunnel: [w600 w601] -> w586
              frame No Error {
                n90 = call "Start Polling Pressure Regulator Status.vi"("error in"=w598, "Polling Interval [ms]"=1000) -> ("error out"=w600:errorcluster)  [unwired: 9 in]
                n91 = call "Wake Purge Strategy Helper Loop.vi"("error in"=w598) -> ()  [unwired: 10 in, 1 out]
              }
              frame Error {
                n92 = call "Wake Connection Helper Loop.vi"("error in"=w602) -> ("error out"=w601:errorcluster)  [unwired: 10 in]
              }
            }
            n93 = Bundle By Name(cluster=w583, "Modbus Config"=w584, "MB_TCP session"=w589) -> (w588:T1)
          }
          frame "Set Anode Inlet Pressure SP" {
            # "Flow Setpoint must be zero to close control valve"
            # "Sets the anode inlet pressure setpoint."
            n94 = Variant To Data(error in=w614, type=T15 {"Anode Inlet Pressure [bar]"=0.0} ("Set Anode Inlet Pressure SP Argument"), Variant=w613) -> (data=w611:T15, error out=w608:errorcluster)
            n95 = Unbundle By Name(w610) -> ("MB_TCP session"=w607:refnum<class "MB_Master_TCP.lvclass">)
            n96 = Unbundle By Name(w611) -> ("Anode Inlet Pressure [bar]"=w606:dbl)
            n97 = call "Write P2setpoint (Channel P2).vi"("error in"=w608, "Value"=w606, "MB_TCP session in"=w607) -> ("error out"=w603:errorcluster, "Value"=→"P2 Setpoint":sgl, "MB session out"=w604:refnum<class "MB_Master_TCP.lvclass">)  [unwired: 6 in]
            n98 = Bundle By Name(cluster=w610, "MB_TCP session"=w604) -> (w609:T1)
          }
          frame "Read Pressure Regulator Status" {
            # "Reads the pressure regulator status."
            n99 = Variant To Data(error in=w625, type=T13 {"Boolean"=FALSE} ("Read Pressure Regulator Status Argument"), Variant=w624) -> (error out=w621:errorcluster)  [unwired: 1 out]
            n100 = Unbundle By Name(w620) -> ("MB_TCP session"=w622:refnum<class "MB_Master_TCP.lvclass">)
            n101 = call "Read measure (Multi-Channel F, P1 and P2).vi"("error in"=w621, "MB_TCP session in"=w622) -> ("error out"=w615:errorcluster, "Fmeasure (F, P1, P2)"=w617:T3, "MB session out"=w616:refnum<class "MB_Master_TCP.lvclass">)  [unwired: 7 in]
            n102 = case shown="Error .." w615 {
              selector: w615 -> [w626 _]
              tunnel: w620 -> [w637 w640]
              tunnel: [w636 w640] -> w619
              tunnel: [w635 w639] -> w618
              tunnel: w617 -> [w634 _]
              tunnel: w616 -> [w632 _]
              frame No Error {
                n103 = call "Read Counter.vi"("error in"=w626, "MB_TCP session in"=w632) -> ("error out"=w633:errorcluster, "Value"=w628:sgl, "MB session out"=w631:refnum<class "MB_Master_TCP.lvclass">)  [unwired: 7 in]
                "Counter In" <- w628
                n104 = call "Anode State Cluster to Map.vi"("Fmeasure (F, P1, P2) in"=w634) -> ("Anode Status Map"=w630:map{string, dbl})  [unwired: 10 in]
                n105 = Insert Into Map(map in=w630, key="stack__anode__h2_counter_in", value=w628) -> (map out=w629:map{string, dbl})  [unwired: 2 out]
                n106 = Bundle By Name(cluster=w637, "MB_TCP session"=w631, "Fmeasure (F, P1, P2)"=w634, "Anode Status Map"=w629) -> (w636:T1)
                n107 = call "Broadcast Anode State.vi"("error in"=w633, "Anode State Map"=w629) -> ("error out"=w635:errorcluster)  [unwired: 9 in]
                "Fmeasure (F, P1, P2)" <- w634
              }
              frame Error {
                n108 = call "Stop Polling Pressure Regulator Status.vi"() -> ("error out"=w638:errorcluster)  [unwired: 11 in]
                n109 = call "Wake Connection Helper Loop.vi"("error in"=w638) -> ("error out"=w639:errorcluster)  [unwired: 10 in]
              }
            }
          }
          frame "Set Pressure Regulator Control Function" {
            # "Sets the pressure regulator control function."
            n110 = Variant To Data(error in=w652, type=T16 {"Function"=enum."Flow"} ("Set Pressure Regulator Control Function Argument"), Variant=w651) -> (data=w649:T16, error out=w648:errorcluster)
            n111 = Unbundle By Name(w644) -> ("MB_TCP session"=w645:refnum<class "MB_Master_TCP.lvclass">)
            n112 = Unbundle By Name(w649) -> ("Function"=w646:T17)
            n113 = call "Write Control Function.vi"("error in"=w648, "Function"=w646, "MB_TCP session in"=w645) -> ("error out"=w647:errorcluster, "Value"=→"Control Function":u16, "MB session out"=w642:refnum<class "MB_Master_TCP.lvclass">)  [unwired: 6 in]
            n114 = Bundle By Name(cluster=w644, "MB_TCP session"=w642) -> (w643:T1)
          }
          frame "Set Anode Inlet Flow SP" {
            # "Sets the anode inlet flow setpoint [slm]."
            n115 = Variant To Data(error in=w664, type=T18 {"Flow SP [slm]"=0.0} ("Set Anode Inlet Flow SP Argument"), Variant=w663) -> (data=w661:T18, error out=w660:errorcluster)
            n116 = Unbundle By Name(w661) -> ("Flow SP [slm]"=w658:dbl)
            n117 = Unbundle By Name(w656) -> ("MB_TCP session"=w657:refnum<class "MB_Master_TCP.lvclass">)
            n118 = call "Write Fsetpoint (Channel F).vi"("error in"=w660, "Value"=w658, "MB_TCP session in"=w657) -> ("error out"=w659:errorcluster, "Value"=w653:sgl, "MB session out"=w654:refnum<class "MB_Master_TCP.lvclass">)  [unwired: 6 in]
            "Value" <- w653
            n119 = Bundle By Name(cluster=w656, "MB_TCP session"=w654, "Flow Rate SP (Valve Shutoff)"=w653) -> (w655:T1)
          }
          frame "Set Anode Inlet Valve State" {
            w666 = u16 0 items=["Observe"=0, "Ignore"=256] ("Obersve or Ignore Safe State")
            # "This code is horrible..."
            # "Sets the anode inlet solenoid valve state."
            n120 = Variant To Data(error in=w677, type=T19 {"Anode Solenoid Valve"=enum."CLOSED"} ("Set Anode Inlet Solenoid Valve State Argument"), Variant=w676) -> (data=w674:T19, error out=w671:errorcluster)
            n121 = Unbundle By Name(w673) -> ("MB_TCP session"=w669:refnum<class "MB_Master_TCP.lvclass">)
            n122 = Unbundle By Name(w674) -> ("Anode Solenoid Valve"=w667:T2)
            n123 = case shown="\"CLOSED\", Default" w667 {
              tunnel: [Valve_State--enum."Close" ("Valve State") Valve_State--enum."Open" ("Valve State")] -> w665
              frame "CLOSED", Default {
              }
              frame "OPEN" {
              }
            }
            n124 = call "Write Shutoff Valve State.vi"("error in"=w671, "Obersve or Ignore Safe State"=w666, "Valve State"=w665, "MB_TCP session in"=w669) -> ("error out"=w670:errorcluster, "MB session out"=w668:refnum<class "MB_Master_TCP.lvclass">)  [unwired: 5 in, 1 out]
            n125 = Bundle By Name(cluster=w673, "MB_TCP session"=w668) -> (w672:T1)
          }
          frame "Set Anode Gas Supply Valve" {
            # "Sets anode gas supply valve."
            n126 = Variant To Data(error in=w692, type=T20 {"Valve State"=enum."CLOSED"} ("Set Anode Gas Supply Valve Argument"), Variant=w691) -> (data=w689:T20, error out=w688:errorcluster)
            n127 = Unbundle By Name(w689) -> ("Valve State"=w682:enum16{"CLOSED", "OPEN"})
            n128 = Unbundle By Name(w685) -> ("DAQmx Task Gas Supply"=w686:refnum<k21>)
            n129 = case shown="\"CLOSED\", Default" w682 {
              tunnel: [FALSE TRUE] -> w681
              frame "CLOSED", Default {
              }
              frame "OPEN" {
              }
            }
            n130 = call-poly <vilib>:"DAQmx Write.vi"("task/channels in"=w686, "data"=w681, "timeout"=1.0, "error in"=w688) -> ("task out"=w683:refnum<k21>, "error out"=w687:errorcluster)  [unwired: 9 in, 1 out]
            n131 = Bundle By Name(cluster=w685, "DAQmx Task Gas Supply"=w683) -> (w684:T1)
          }
          frame "Set Purge Valve" {
            # "Sets the purge valve open or closed."
            n132 = Variant To Data(error in=w705, type=T21 {"Valve State"=enum."CLOSED"} ("Set Purge Valve Argument"), Variant=w704) -> (data=w702:T21, error out=w697:errorcluster)
            n133 = Unbundle By Name(w702) -> ("Valve State"=w701:enum16{"CLOSED", "OPEN"})
            n134 = Unbundle By Name(w700) -> ("Purge Strategy"=w699:T5)
            n135 = case shown="\"OPEN\"" w701 {
              tunnel: [Purge_Strategy--enum."FORCE OFF" ("Strategy") Purge_Strategy--enum."FORCE ON" ("Strategy")] -> w696
              frame "CLOSED", Default {
              }
              frame "OPEN" {
              }
            }
            n136 = Bundle By Name(cluster=w699, "Strategy"=w696) -> (w695:T5)
            n137 = call "Update Purge Strategy Settings.vi"("error in"=w697, "Purge Settings"=w695) -> ("error out"=w698:errorcluster)  [unwired: 9 in]
          }
          frame "Set Purge Strategy" {
            # "Sets the purge strategy."
            n138 = Variant To Data(error in=w716, type=T22 {"Purge Controller"={"Strategy"=enum."FORCE OFF", "Purge Interval [s]"=30.0, "Purge Duration [s]"=1.0}} ("Set Purge Strategy Argument"), Variant=w715) -> (data=w713:T22, error out=w710:errorcluster)
            n139 = Unbundle By Name(w713) -> ("Purge Controller"=w708:T5)
            n140 = Bundle By Name(cluster=w712, "Purge Strategy"=w708) -> (w711:T1)
            n141 = call "Update Purge Strategy Settings.vi"("error in"=w710, "Purge Settings"=w708) -> ("error out"=w709:errorcluster)  [unwired: 9 in]
          }
          frame "Wake Purge Helper Loop" {
            # "Wake Purge Helper Loop."
            n142 = Variant To Data(error in=w722, type=T23 {"Boolean"=FALSE} ("Wake Purge Helper Loop Argument"), Variant=w720) -> (error out=w718:errorcluster)  [unwired: 1 out]
            n143 = call "Wake Purge Strategy Helper Loop.vi"("error in"=w718) -> ("error out"=w717:errorcluster)  [unwired: 10 in]
          }
          frame "Reset Counter" {
            # "Resets the counter."
            n144 = Variant To Data(error in=w732, type=T24 {"Boolean"=FALSE} ("Reset Counter Argument"), Variant=w731) -> (error out=w729:errorcluster)  [unwired: 1 out]
            n145 = Unbundle By Name(w725) -> ("MB_TCP session"=w726:refnum<class "MB_Master_TCP.lvclass">)
            n146 = call "Write Reset.vi"("error in"=w729, "Reset Arguments"=T29."Reset counter (all)", "MB_TCP session in"=w726) -> ("error out"=w728:errorcluster, "MB session out"=w723:refnum<class "MB_Master_TCP.lvclass">)  [unwired: 7 in]
            n147 = Bundle By Name(cluster=w725, "MB_TCP session"=w723) -> (w724:T1)
          }
          frame "Start H2 Sensor Measurement" {
            # "#DQMH_CodeNeeded\n1. Configure this Message Case for handling the \"Start H2 Sensor Measurement\" message.\n2. Delete or edit this label when done."
            # "Starts the H2 sensor measurement."
            n148 = Variant To Data(error in=w738, type=T25 {"Boolean"=FALSE} ("Start H2 Sensor Measurement Argument"), Variant=w736) -> (error out=w734:errorcluster)  [unwired: 1 out]
            n149 = call "Wake H2 Sensor Loop.vi"("error in"=w734) -> ("error out"=w733:errorcluster)  [unwired: 10 in]
          }
          frame "Stop H2 Sensor Measurement" {
            # "Stops the H2 sensor measurement."
            n150 = Variant To Data(error in=w744, type=T26 {"Boolean"=FALSE} ("Stop H2 Sensor Measurement Argument"), Variant=w742) -> (error out=w740:errorcluster)  [unwired: 1 out]
            n151 = call "Sleep H2 Sensor Loop.vi"("error in"=w740) -> ("error out"=w739:errorcluster)  [unwired: 10 in]
          }
          frame "---Copy This Frame---" {
            # "Duplicate this frame when creating new messages.  Change this comment in the duplicated frame to describe this message."
            n152 = Merge Errors(w747) -> (w745:errorcluster)
          }
          frame "--- Exit and Error Handling---" {
            # "Separator - The following cases handle errors and exit messages."
            n153 = Merge Errors(w750) -> (w748:errorcluster)
          }
          frame "Simulate MHL Error" {
            # "Simulate an error occurring at the MHL"
            n154 = call "Module Name--constant.vi"() -> ("Module Name"=w752:string)  [unwired: 11 in]
            n155 = xnode "Error Ring"("parameter 0"=w752) -> ("error out"=w751:errorcluster)
            n156 = Merge Errors(w755, w751) -> (w753:errorcluster)
          }
          frame "Error" {
            # "#CodeRecommended - If you ever change the name of this \"Error\" message, you'll need to update the name in the Check Loop Error.vi as well."
            # "#CodeRecommended - If the module is running in standalone mode (External Launch = FALSE), this code will pop up an error dialog and call the 'Exit' message if an error occurs. Add more fine-grained error handling here."
            # "Error - Check the error message data and respond accordingly. This message is sent by the \"Error Handler\" VIs at the end of each loop in this application."
            n157 = property on="Property Node" class="Module Admin"(reference=w765) -> ("Accessors:External Launch"=w764:bool)  [unwired: 1 in, 2 out]
            n158 = Variant To Data(error in=w772, type=errorcluster {"status"=FALSE, "code"=0, "source"=""} ("error constant"), Variant=w770) -> (data=w773:errorcluster, error out=w768:errorcluster)
            n159 = call "Error Reported.vi"("Error"=w773) -> ()  [unwired: 10 in, 1 out]
            n160 = case shown="True" w764 {
              tunnel: [w778 _] -> w767
              tunnel: w766 -> [w777 _]
              tunnel: w773 -> [w774 _]
              frame False {
                # "If the module is running standalone, then pop up an error dialog and call the \"Exit\" message."
                n161 = call <vilib>:"Simple Error Handler.vi"("error in (no error)"=w774) -> ()  [unwired: 4 in, 5 out]
                n162 = call-poly <vilib>:"Delacor_lib_QMH_Enqueue Message (poly).vi"("Priority Message? (F)"=TRUE, "Message"="Exit", "Message Queue in"=w777) -> ("error out"=w778:errorcluster)  [unwired: 7 in, 1 out]
              }
              frame True {
                # "If the module was launched externally, calling the Error Reported broadcast VI is the only action performed by the \"Error\" message. The module's caller can then process the error appropriately."
              }
            }
            n163 = Merge Errors(w768, w767) -> (w763:errorcluster)
            n164 = local write "error out"(w763) -> ()
          }
          frame "Confirm Quit" {
            # "#CodeNeeded - If you want to provide an \"Are you sure\" dialog (or some other notification) before the application exits, place that code here. This message is typically sent from a Panel Close? event."
            # "Confirm Quit - Message that can confirm whether or not the user wants to exit the application."
            n165 = call-poly <vilib>:"Delacor_lib_QMH_Enqueue Message (poly).vi"("Priority Message? (F)"=TRUE, "error in"=w785, "Message"="Exit", "Message Queue in"=w781) -> ("error out"=w782:errorcluster)  [unwired: 6 in, 1 out]
            n166 = Merge Errors(w782) -> (w783:errorcluster)
          }
          frame "Exit" {
            w792 = u16 0 items=["Observe"=0, "Ignore"=256] ("Obersve or Ignore Safe State")
            w798 = 91  # 91: not all Exit messages will have an argument
            w803 = TRUE  # Stop the VI
            # "Release the message queue reference"
            # "#CodeNeeded - Add any required cleanup code here"
            # "Exit - Exit the application."
            n167 = Variant To Data(error in=w806, type=T14 {"Origin"="", "Exit via Stop Module Req?"=FALSE, "Wait for Module to stop?"=FALSE} ("Stop Argument"), Variant=w800) -> (data=w796:T14, error out=w799:errorcluster)
            n168 = call <vilib>:"Clear Errors.vi"("error in (no error)"=w799, "specific error code to clear (0: all)"=w798) -> ("error out"=w805:errorcluster)  [unwired: 4 in, 1 out]
            n169 = Unbundle By Name(w793) -> ("MB_TCP session"=w790:refnum<class "MB_Master_TCP.lvclass">)
            n170 = call-dynamic "Delacor_lib_QMH_Release Message Queue.vi"("error in"=w805, "Message Queue"=w804) -> ("error out"=w802:errorcluster)  [unwired: 9 in]
            n171 = call "Write Shutoff Valve State.vi"("Obersve or Ignore Safe State"=w792, "Valve State"=Valve_State--enum."Close", "MB_TCP session in"=w790) -> ("error out"=w788:errorcluster, "MB session out"=w789:refnum<class "MB_Master_TCP.lvclass">)  [unwired: 6 in, 1 out]
            n172 = call "Modbus TCP Close.vi"("error in (no error)"=w788, "MB session in"=w789) -> ("error out"=w787:errorcluster)  [unwired: 9 in]
            n173 = call "Handle Exit.vi"("Stop Argument"=w796, "Admin in"=w795) -> ("error out"=w794:errorcluster)  [unwired: 8 in, 1 out]
            n174 = call <vilib>:"Clear Errors.vi"("error in (no error)"=w787) -> ("error out"=w786:errorcluster)  [unwired: 5 in, 1 out]
            n175 = Merge Errors(w794, w786, w802) -> (w801:errorcluster)
            n176 = call "Error Reported.vi"("Error"=w801) -> ()  [unwired: 10 in, 1 out]
          }
          frame Default {
            # "'Default' case only runs if there is a message that isn't defined in any of the other cases.  Output a programming error."
            n177 = call "Module Name--constant.vi"() -> ("Module Name"=w807:string)  [unwired: 11 in]
            n178 = xnode "Error Ring"("parameter 0"=w808, "parameter 1"=w807) -> ("error out"=w809:errorcluster)
          }
        }
        "Data Cluster" <- w535
        n179 = call-dynamic "Delacor_lib_QMH_Error Handler - Message Handling Loop.vi"("error in"=w537, "Message Queue in"=w528) -> ("dup error in"=w527:errorcluster)  [unwired: 8 in, 1 out]
      }
      n180 = while {
        tunnel: w61 -> [w351]
        shift-right: [w349] -> w64
        shift-left: w62 -> [w350]
        tunnel: [w345] -> w60
        tunnel: w58 -> [w344]
        tunnel: w57 -> [w343]
        shift-right: [w341] -> w55
        shift-left: w56 -> [w342]
        stop <- w347 stop-if-true
        # "Event Handling Loop"
        n181 = event "DQMH_EVENT_MAIN" shown="[21] <Anode Request Events.Stop H2 Sensor Measurement>: User Event" {
          selector: w350 -> [_ _ _ _ _ _ _ _ _ _ _ _ _ _ _ _ _ _ _ _ _ _]
          dyn-events: [_ _ _ _ _ _ _ _ _ _ _ _ _ _ _ _ _ _ _ _ _ _] -> w349
          timeout: _ -> [_ _ _ _ _ _ _ _ _ _ _ _ _ _ _ _ _ _ _ _ _ _]
          tunnel: [_ _ _ _ _ _ TRUE ("Discard?") _ _ _ _ _ _ _ _ _ _ _ _ _ _ _] -> w347
          tunnel: w351 -> [w355 w367 w371 w374 w378 w383 w395 w405 w412 w429 w437 w445 w453 w461 w469 w477 w485 w493 w501 w509 w517 w525]
          tunnel: [w354 w364 w369 _ w377 w380 w389 w401 w411 w422 w431 w438 w446 w454 w462 w470 w478 w486 w494 w502 w510 w518] -> w348
          tunnel: [w355 w366 w371 w374 w378 w382 w394 w405 w410 w427 w435 w443 w451 w459 w467 w475 w483 w491 w499 w507 w515 w523] -> w346
          tunnel: w344 -> [_ _ _ _ _ _ _ _ w409 _ _ _ _ _ _ _ _ _ _ _ _ _]
          tunnel: w343 -> [_ _ _ _ _ _ _ w400 _ _ _ _ _ _ _ _ _ _ _ _ _ _]
          tunnel: w342 -> [w352 w363 w370 w373 w375 w379 w384 w404 w407 w428 w436 w444 w452 w460 w468 w476 w484 w492 w500 w508 w516 w524]
          tunnel: [w352 w363 w370 w373 w375 w379 w384 w399 w406 w428 w436 w444 w452 w460 w468 w476 w484 w492 w500 w508 w516 w524] -> w341
          event "Simulate EHL Error": Value Change {
            # "This case simulates an error being generated at the EHL"
            n182 = event-data() -> ()  [unwired: 1 in, 1 out]
            n183 = call "Module Name--constant.vi"() -> ("Module Name"=w353:string)  [unwired: 11 in]
            n184 = xnode "Error Ring"("parameter 0"=w353) -> ("error out"=w354:errorcluster)
          }
          event "Simulate MHL Error": Value Change {
            # "This case simulates an error being generated at the EHL"
            n185 = event-data() -> ()  [unwired: 1 in, 1 out]
            n186 = call-poly <vilib>:"Delacor_lib_QMH_Enqueue Message (poly).vi"("Message"="Simulate MHL Error", "Message Queue in"=w367) -> ("error out"=w364:errorcluster, "Message Queue out"=w366:refnum<class "Delacor_lib_QMH_Message Queue.lvclass">)  [unwired: 8 in]
          }
          event User Event {
            # "Another Module called the \"Show Panel\" API Method."
            n187 = event-data() -> ()  [unwired: 1 in, 1 out]
            n188 = call <vilib>:"Show.vi"("Panel in"=w370) -> ("Error Out"=w369:errorcluster)  [unwired: 10 in]
            n189 = call "Status Updated.vi"("Status"="Panel shown." ("format string")) -> ()  [unwired: 10 in, 1 out]
          }
          event User Event {
            # "Another Module called the \"Hide Panel\" API Method."
            n190 = event-data() -> ()  [unwired: 1 in, 1 out]
            n191 = call <vilib>:"Hide.vi"("Panel In"=w373) -> ()  [unwired: 10 in, 1 out]
            n192 = call "Status Updated.vi"("Status"="Panel hidden." ("format string")) -> ()  [unwired: 10 in, 1 out]
          }
          event User Event {
            # "Another Module called the \"Get Module Execution Status\" API Method."
            n193 = event-data() -> ()  [unwired: 1 in, 1 out]
            n194 = call "Update Module Execution Status.vi"("Running?"=TRUE) -> ("error out"=w377:errorcluster)  [unwired: 10 in]
          }
          event User Event {
            # "Another Module called the \"Show Diagram\" API Method."
            n195 = event-data() -> ()  [unwired: 1 in, 1 out]
            n196 = call-poly <vilib>:"Delacor_lib_QMH_Enqueue Message (poly).vi"("Message"="Show Diagram", "Message Queue in"=w383) -> ("error out"=w380:errorcluster, "Message Queue out"=w382:refnum<class "Delacor_lib_QMH_Message Queue.lvclass">)  [unwired: 8 in]
          }
          event User Event {
            # "The Stop Module Event can get fired from the Exit message in the MHL. The queue gets destroyed in that case. If the queue no longer exists, the Enqueue Exit as a priority message will return error 1. It is safe to ignore, because the module is already exiting."
            # "Another Module called the \"Stop Module\" API Method  or the Message Handling Loop below."
            n197 = event-data() -> ("Origin"=w393:string, "Exit via Stop Module Req?"=w387:bool, "Wait for Module to stop?"=w386:bool)  [unwired: 1 in]
            n198 = call <vilib>:"Hide.vi"("Panel In"=w384) -> ()  [unwired: 10 in, 1 out]
            n199 = local write "Status"(w393) -> ()
            n200 = Bundle By Name(cluster=T14 {"Origin"="", "Exit via Stop Module Req?"=FALSE, "Wait for Module to stop?"=FALSE} ("Stop Argument"), "Exit via Stop Module Req?"=w387, "Wait for Module to stop?"=w386) -> (w385:T14)
            n201 = call-poly <vilib>:"Delacor_lib_QMH_Enqueue Message (poly).vi"("Priority Message? (F)"=TRUE, "Message Data"=w385, "Message"="Exit", "Message Queue in"=w395) -> ("error out"=w390:errorcluster, "Message Queue out"=w394:refnum<class "Delacor_lib_QMH_Message Queue.lvclass">)  [unwired: 6 in]
            n202 = call <vilib>:"Clear Errors.vi"("error in (no error)"=w390, "specific error code to clear (0: all)"=1) -> ("error out"=w389:errorcluster)  [unwired: 4 in, 1 out]
          }
          event User Event {
            # "Another Module called the \"Change Panel\" API Method."
            n203 = event-data() -> ("New Panel"=w403:refnum<class "Panel.lvclass">)  [unwired: 1 in]
            n204 = call-dynamic <vilib>:"Close.vi"("Panel In"=w404) -> ("Error Out"=w402:errorcluster)  [unwired: 10 in]
            n205 = call <vilib>:"Initialize.vi"("error in (no error)"=w402, "My Helper in"=w400, "Panel In"=w403) -> ("error out"=w401:errorcluster, "Panel Out"=w399:refnum<class "Panel.lvclass">)  [unwired: 6 in, 1 out]
            n206 = call "Status Updated.vi"("Status"="Panel changed.") -> ()  [unwired: 10 in, 1 out]
          }
          event Panel Close? {
            w413 = TRUE  # Discard the event so the 'Confirm Quit' message has a chance to run.
            # "If launched externally, closing the panel doesn't quit the VI."
            # "Send the 'Confirm Quit' message if the user closes the panel of the VI."
            n207 = event-data() -> ()  [unwired: 1 in, 1 out]
            n208 = property on="Property Node" class="Module Admin"(reference=w409) -> ("Accessors:External Launch"=w408:bool)  [unwired: 1 in, 2 out]
            n209 = case shown="True" w408 {
              tunnel: w412 -> [w418 w421]
              tunnel: [w417 w419] -> w411
              tunnel: [w416 w421] -> w410
              tunnel: w407 -> [w414 w420]
              tunnel: [w414 w420] -> w406
              frame False {
                n210 = call-poly <vilib>:"Delacor_lib_QMH_Enqueue Message (poly).vi"("Message"="Confirm Quit", "Message Queue in"=w418) -> ("error out"=w417:errorcluster, "Message Queue out"=w416:refnum<class "Delacor_lib_QMH_Message Queue.lvclass">)  [unwired: 8 in]
              }
              frame True {
                n211 = call <vilib>:"Hide.vi"("Panel In"=w420) -> ("Error Out"=w419:errorcluster)  [unwired: 10 in]
              }
            }
            n212 = event-data ("Event Filter Node")("Discard?"=w413) -> ()  [unwired: 1 in, 1 out]
          }
          event User Event {
            # "Another Module called the \"Set Anode Inlet Pressure SP\" API Method."
            n213 = event-data() -> ("Anode Inlet Pressure [bar]"=w423:dbl)  [unwired: 1 in]
            n214 = Bundle(cluster=T15 {"Anode Inlet Pressure [bar]"=0.0} ("Set Anode Inlet Pressure SP Argument"), "Anode Inlet Pressure [bar]"=w423) -> (w424:T15)
            n215 = call-poly <vilib>:"Delacor_lib_QMH_Enqueue Message (poly).vi"("Message Data"=w424, "Message"="Set Anode Inlet Pressure SP", "Message Queue in"=w429) -> ("error out"=w422:errorcluster, "Message Queue out"=w427:refnum<class "Delacor_lib_QMH_Message Queue.lvclass">)  [unwired: 7 in]
          }
          event User Event {
            # "Another Module called the \"Initialise Pressure Regulator Interface\" API Method."
            n216 = event-data() -> ("Modbus Config"=w430:T4)  [unwired: 1 in]
            n217 = Bundle(cluster=T12 {"Modbus Config"={"IP Address"="localhost", "Port (502)"=502, "Slave ID (255)"=16, "Timeout (10000)"=10000}} ("Initialise Pressure Regulator Interface Argument"), "Modbus Config"=w430) -> (w432:T12)
            n218 = call-poly <vilib>:"Delacor_lib_QMH_Enqueue Message (poly).vi"("Message Data"=w432, "Message"="Initialise Pressure Regulator Interface", "Message Queue in"=w437) -> ("error out"=w431:errorcluster, "Message Queue out"=w435:refnum<class "Delacor_lib_QMH_Message Queue.lvclass">)  [unwired: 7 in]
          }
          event User Event {
            # "Another Module called the \"Read Pressure Regulator Status\" API Method."
            n219 = event-data() -> ("Boolean"=w439:bool)  [unwired: 1 in]
            n220 = Bundle(cluster=T13 {"Boolean"=FALSE} ("Read Pressure Regulator Status Argument"), "Boolean"=w439) -> (w440:T13)
            n221 = call-poly <vilib>:"Delacor_lib_QMH_Enqueue Message (poly).vi"("Message Data"=w440, "Message"="Read Pressure Regulator Status", "Message Queue in"=w445) -> ("error out"=w438:errorcluster, "Message Queue out"=w443:refnum<class "Delacor_lib_QMH_Message Queue.lvclass">)  [unwired: 7 in]
          }
          event User Event {
            # "Another Module called the \"Set Pressure Regulator Control Function\" API Method."
            n222 = event-data() -> ("Function"=w447:T17)  [unwired: 1 in]
            n223 = Bundle(cluster=T16 {"Function"=enum."Flow"} ("Set Pressure Regulator Control Function Argument"), "Function"=w447) -> (w448:T16)
            n224 = call-poly <vilib>:"Delacor_lib_QMH_Enqueue Message (poly).vi"("Message Data"=w448, "Message"="Set Pressure Regulator Control Function", "Message Queue in"=w453) -> ("error out"=w446:errorcluster, "Message Queue out"=w451:refnum<class "Delacor_lib_QMH_Message Queue.lvclass">)  [unwired: 7 in]
          }
          event User Event {
            # "Another Module called the \"Set Anode Inlet Flow SP\" API Method."
            n225 = event-data() -> ("Flow SP [slm]"=w455:dbl)  [unwired: 1 in]
            n226 = Bundle(cluster=T18 {"Flow SP [slm]"=0.0} ("Set Anode Inlet Flow SP Argument"), "Flow SP [slm]"=w455) -> (w456:T18)
            n227 = call-poly <vilib>:"Delacor_lib_QMH_Enqueue Message (poly).vi"("Message Data"=w456, "Message"="Set Anode Inlet Flow SP", "Message Queue in"=w461) -> ("error out"=w454:errorcluster, "Message Queue out"=w459:refnum<class "Delacor_lib_QMH_Message Queue.lvclass">)  [unwired: 7 in]
          }
          event User Event {
            # "Another Module called the \"Set Anode Inlet Solenoid Valve State\" API Method."
            n228 = event-data() -> ("Anode Solenoid Valve"=w463:T2)  [unwired: 1 in]
            n229 = Bundle(cluster=T19 {"Anode Solenoid Valve"=enum."CLOSED"} ("Set Anode Inlet Solenoid Valve State Argument"), "Anode Solenoid Valve"=w463) -> (w464:T19)
            n230 = call-poly <vilib>:"Delacor_lib_QMH_Enqueue Message (poly).vi"("Message Data"=w464, "Message"="Set Anode Inlet Valve State", "Message Queue in"=w469) -> ("error out"=w462:errorcluster, "Message Queue out"=w467:refnum<class "Delacor_lib_QMH_Message Queue.lvclass">)  [unwired: 7 in]
          }
          event User Event {
            # "Another Module called the \"Set Anode Gas Supply Valve\" API Method."
            n231 = event-data() -> ("Valve State"=w471:enum16{"CLOSED", "OPEN"})  [unwired: 1 in]
            n232 = Bundle(cluster=T20 {"Valve State"=enum."CLOSED"} ("Set Anode Gas Supply Valve Argument"), "Valve State"=w471) -> (w472:T20)
            n233 = call-poly <vilib>:"Delacor_lib_QMH_Enqueue Message (poly).vi"("Message Data"=w472, "Message"="Set Anode Gas Supply Valve", "Message Queue in"=w477) -> ("error out"=w470:errorcluster, "Message Queue out"=w475:refnum<class "Delacor_lib_QMH_Message Queue.lvclass">)  [unwired: 7 in]
          }
          event User Event {
            # "Another Module called the \"Set Purge Valve\" API Method."
            n234 = event-data() -> ("Valve State"=w479:enum16{"CLOSED", "OPEN"})  [unwired: 1 in]
            n235 = Bundle(cluster=T21 {"Valve State"=enum."CLOSED"} ("Set Purge Valve Argument"), "Valve State"=w479) -> (w480:T21)
            n236 = call-poly <vilib>:"Delacor_lib_QMH_Enqueue Message (poly).vi"("Message Data"=w480, "Message"="Set Purge Valve", "Message Queue in"=w485) -> ("error out"=w478:errorcluster, "Message Queue out"=w483:refnum<class "Delacor_lib_QMH_Message Queue.lvclass">)  [unwired: 7 in]
          }
          event User Event {
            # "Another Module called the \"Set Purge Strategy\" API Method."
            n237 = event-data() -> ("Purge Controller"=w487:T5)  [unwired: 1 in]
            n238 = Bundle(cluster=T22 {"Purge Controller"={"Strategy"=enum."FORCE OFF", "Purge Interval [s]"=30.0, "Purge Duration [s]"=1.0}} ("Set Purge Strategy Argument"), "Purge Controller"=w487) -> (w488:T22)
            n239 = call-poly <vilib>:"Delacor_lib_QMH_Enqueue Message (poly).vi"("Message Data"=w488, "Message"="Set Purge Strategy", "Message Queue in"=w493) -> ("error out"=w486:errorcluster, "Message Queue out"=w491:refnum<class "Delacor_lib_QMH_Message Queue.lvclass">)  [unwired: 7 in]
          }
          event User Event {
            # "Another Module called the \"Wake Purge Helper Loop\" API Method."
            n240 = event-data() -> ("Boolean"=w495:bool)  [unwired: 1 in]
            n241 = Bundle(cluster=T23 {"Boolean"=FALSE} ("Wake Purge Helper Loop Argument"), "Boolean"=w495) -> (w496:T23)
            n242 = call-poly <vilib>:"Delacor_lib_QMH_Enqueue Message (poly).vi"("Message Data"=w496, "Message"="Wake Purge Helper Loop", "Message Queue in"=w501) -> ("error out"=w494:errorcluster, "Message Queue out"=w499:refnum<class "Delacor_lib_QMH_Message Queue.lvclass">)  [unwired: 7 in]
          }
          event User Event {
            # "Another Module called the \"Reset Counter\" API Method."
            n243 = event-data() -> ("Boolean"=w503:bool)  [unwired: 1 in]
            n244 = Bundle(cluster=T24 {"Boolean"=FALSE} ("Reset Counter Argument"), "Boolean"=w503) -> (w504:T24)
            n245 = call-poly <vilib>:"Delacor_lib_QMH_Enqueue Message (poly).vi"("Message Data"=w504, "Message"="Reset Counter", "Message Queue in"=w509) -> ("error out"=w502:errorcluster, "Message Queue out"=w507:refnum<class "Delacor_lib_QMH_Message Queue.lvclass">)  [unwired: 7 in]
          }
          event User Event {
            # "Another Module called the \"Start H2 Sensor Measurement\" API Method."
            n246 = event-data() -> ("Boolean"=w511:bool)  [unwired: 1 in]
            n247 = Bundle(cluster=T25 {"Boolean"=FALSE} ("Start H2 Sensor Measurement Argument"), "Boolean"=w511) -> (w512:T25)
            n248 = call-poly <vilib>:"Delacor_lib_QMH_Enqueue Message (poly).vi"("Message Data"=w512, "Message"="Start H2 Sensor Measurement", "Message Queue in"=w517) -> ("error out"=w510:errorcluster, "Message Queue out"=w515:refnum<class "Delacor_lib_QMH_Message Queue.lvclass">)  [unwired: 7 in]
          }
          event User Event {
            # "Another Module called the \"Stop H2 Sensor Measurement\" API Method."
            n249 = event-data() -> ("Boolean"=w519:bool)  [unwired: 1 in]
            n250 = Bundle(cluster=T26 {"Boolean"=FALSE} ("Stop H2 Sensor Measurement Argument"), "Boolean"=w519) -> (w520:T26)
            n251 = call-poly <vilib>:"Delacor_lib_QMH_Enqueue Message (poly).vi"("Message Data"=w520, "Message"="Stop H2 Sensor Measurement", "Message Queue in"=w525) -> ("error out"=w518:errorcluster, "Message Queue out"=w523:refnum<class "Delacor_lib_QMH_Message Queue.lvclass">)  [unwired: 7 in]
          }
        }
        n252 = call-dynamic "Delacor_lib_QMH_Error Handler - Event Handling Loop.vi"("error in"=w348, "Message Queue in"=w346) -> ("dup error in"=w345:errorcluster)  [unwired: 8 in, 1 out]
      }
      n253 = while "DQMH_HELPER_LOOP" {
        shift-right: [w328] -> _
        shift-left: -1 -> [w327]
        shift-right: [w325] -> w53
        shift-left: w52 -> [w326]
        tunnel: w61 -> [w322]
        stop <- w324 stop-if-true
        w321 = "Pressure Regulator Status Helper Loop"  # DQMH_HELPER_LOOP_NAME
        # "Pressure Regulator Status Helper Loop"
        n254 = event "DQMH_HELPER_EVENT_STRUCTURE" shown="[0] Timeout" {
          selector: w326 -> [_ _ _ _]
          dyn-events: [_ _ _ _] -> w325
          timeout: w327 -> [_ _ _ _]
          tunnel: w327 -> [w335 w338 _ _]
          tunnel: [w335 w338 w339 -1] -> w328
          tunnel: [_ TRUE _ _] -> w324
          tunnel: [w330 errorcluster {"status"=FALSE, "code"=0, "source"=""} ("error constant") _ _] -> w323
          tunnel: w322 -> [w329 _ _ _]
          event Timeout {
            n255 = event-data() -> ()  [unwired: 1 in, 1 out]
            n256 = Bundle(cluster=T13 {"Boolean"=FALSE} ("Read Pressure Regulator Status Argument"), "Boolean"=TRUE) -> (w333:T13)
            n257 = call-poly <vilib>:"Delacor_lib_QMH_Enqueue Message (poly).vi"("Message Data"=w333, "Message"="Read Pressure Regulator Status", "Message Queue in"=w329) -> ("error out"=w330:errorcluster)  [unwired: 7 in, 1 out]
          }
          event User Event {
            n258 = event-data() -> ()  [unwired: 1 in, 1 out]
          }
          event User Event {
            # "Another Module called the \"Read Pressure Regulator Status\" API Method."
            n259 = event-data() -> ("Polling Interval [ms]"=w339:i32)  [unwired: 1 in]
          }
          event User Event {
            # "Another Module called the \"Stop Polling Pressure Regulator Status\" API Method."
            n260 = event-data() -> ()  [unwired: 1 in, 1 out]
          }
        }
        n261 = call-dynamic "Delacor_lib_QMH_Error Handler - Helper Loop.vi"("Error Debug"=w321, "error in"=w323, "Message Queue in"=w322) -> ()  [unwired: 7 in, 2 out]
      }
      n262 = while "DQMH_HELPER_LOOP" {
        shift-right: [w304] -> _
        shift-left: -1 -> [w303]
        shift-right: [w301] -> w49
        shift-left: w48 -> [w302]
        tunnel: w61 -> [w298]
        stop <- w300 stop-if-true
        w297 = "Wake Connection Helper Loop"  # DQMH_HELPER_LOOP_NAME
        # "Wake Connection Helper Loop"
        n263 = event "DQMH_HELPER_EVENT_STRUCTURE" shown="[2] <Anode Request Events.Private.Wake Connection Helper Loop>: User Event" {
          selector: w302 -> [_ _ _]
          dyn-events: [_ _ _] -> w301
          timeout: w303 -> [_ _ _]
          tunnel: w303 -> [w305 w308 w313]
          tunnel: [w305 w308 w313] -> w304
          tunnel: [_ TRUE _] -> w300
          tunnel: [_ errorcluster {"status"=FALSE, "code"=0, "source"=""} ("error constant") _] -> w299
          tunnel: w298 -> [_ _ w310]
          event Timeout {
            n264 = event-data() -> ()  [unwired: 1 in, 1 out]
          }
          event User Event {
            n265 = event-data() -> ()  [unwired: 1 in, 1 out]
          }
          event User Event {
            # "This module called the \"Private.Wake Connection Helper Loop\" private request."
            n266 = event-data() -> ()  [unwired: 1 in, 1 out]
            n267 = local read "Data Cluster"() -> (w309:T1)
            n268 = Wait (ms)(milliseconds to wait=u32 1000) -> (millisecond timer value=w311:u32)
            n269 = flat-sequence {
              tunnel: w311 -> [_]
              tunnel: w310 -> [w319]
              tunnel: [w318] -> _
              tunnel: w309 -> [w317]
              frame #0 {
                n270 = Unbundle By Name(w317) -> ("Modbus Config"=w315:T4)
                n271 = Bundle By Name(cluster=T12 {"Modbus Config"={"IP Address"="localhost", "Port (502)"=502, "Slave ID (255)"=16, "Timeout (10000)"=10000}} ("Initialise Pressure Regulator Interface Argument"), "Modbus Config"=w315) -> (w314:T12)
                n272 = call-poly <vilib>:"Delacor_lib_QMH_Enqueue Message (poly).vi"("Message Data"=w314, "Message"="Initialise Pressure Regulator Interface", "Message Queue in"=w319) -> ("error out"=w318:errorcluster)  [unwired: 7 in, 1 out]
              }
            }
          }
        }
        n273 = call-dynamic "Delacor_lib_QMH_Error Handler - Helper Loop.vi"("Error Debug"=w297, "error in"=w299, "Message Queue in"=w298) -> ()  [unwired: 7 in, 2 out]
      }
      n274 = while "DQMH_HELPER_LOOP" {
        shift-right: [w252] -> _
        shift-left: -1 -> [w251]
        shift-right: [w249] -> w46
        shift-left: w45 -> [w250]
        tunnel: w61 -> [w246]
        shift-right: [w244] -> _
        shift-left: _ -> [w243]
        shift-right: [w242] -> _
        shift-left: _ -> [w241]
        shift-right: [w240] -> _
        shift-left: _ -> [w239]
        shift-right: [w238] -> _
        shift-left: _ -> [w237]
        tunnel: w38 -> [w236]
        stop <- w248 stop-if-true
        w245 = "Purge Strategy Helper Loop"  # DQMH_HELPER_LOOP_NAME
        # "Purge Strategy Helper Loop"
        n275 = event "DQMH_HELPER_EVENT_STRUCTURE" shown="[0] Timeout" {
          selector: w250 -> [_ _ _ _ _]
          dyn-events: [_ _ _ _ _] -> w249
          timeout: w251 -> [_ _ _ _ _]
          tunnel: w251 -> [w265 w278 _ w286 w296]
          tunnel: [w265 w278 100 w286 w296] -> w252
          tunnel: [_ TRUE _ _ _] -> w248
          tunnel: [_ errorcluster {"status"=FALSE, "code"=0, "source"=""} ("error constant") _ _ _] -> w247
          tunnel: w246 -> [_ _ _ _ _]
          tunnel: [w264 _ _ w283 w295] -> w244
          tunnel: w243 -> [w263 _ _ w283 w294]
          tunnel: [w261 w271 w280 w284 w288] -> w242
          tunnel: w241 -> [w260 w269 _ w284 w293]
          tunnel: [w257 _ w279 w285 w292] -> w240
          tunnel: w239 -> [w257 _ _ _ w291]
          tunnel: [w254 w272 _ _ w290] -> w238
          tunnel: w237 -> [w256 w273 _ _ w289]
          tunnel: w236 -> [_ _ _ _ w287]
          event Timeout {
            n276 = event-data() -> ()  [unwired: 1 in, 1 out]
            n277 = call "Anode Purge Logic.vi"("Purge Strategy"=w257, "Purge State in"=w263) -> ("Valve State"=w258:enum16{"CLOSED", "OPEN"}, "Purge State out"=w264:T31)  [unwired: 8 in]
            n278 = case shown="\"OPEN\"" w258 {
              tunnel: [FALSE TRUE] -> w259
              frame "CLOSED", Default {
              }
              frame "OPEN" {
              }
            }
            n279 = call-poly <vilib>:"DAQmx Write.vi"("task/channels in"=w260, "auto start"=TRUE, "data"=w259, "timeout"=1.0, "error in"=w256) -> ("task out"=w261:refnum<k21>, "error out"=w255:errorcluster)  [unwired: 8 in, 1 out]
            n280 = call <userlib>:"Clear All Errors__ogtk.vi"("Error In"=w255) -> ("Error Out"=w254:errorcluster)  [unwired: 3 in]
          }
          event User Event {
            # "Close valve on shutdown"
            n281 = event-data() -> ()  [unwired: 1 in, 1 out]
            n282 = call-poly <vilib>:"DAQmx Write.vi"("task/channels in"=w269, "auto start"=TRUE, "data"=FALSE, "timeout"=1.0, "error in"=w273) -> ("task out"=w271:refnum<k21>, "error out"=w274:errorcluster)  [unwired: 8 in, 1 out]
            n283 = call <userlib>:"Clear All Errors__ogtk.vi"("Error In"=w274) -> ("Error Out"=w272:errorcluster)  [unwired: 3 in]
          }
          event User Event {
            # "This module called the \"Private.Wake Purge Strategy Helper Loop\" private request."
            n284 = event-data() -> ()  [unwired: 1 in, 1 out]
            n285 = local read "Data Cluster"() -> (w281:T1)
            n286 = Unbundle By Name(w281) -> ("DAQmx Task Purge Valve"=w280:refnum<k21>, "Purge Strategy"=w279:T5)
          }
          event User Event {
            # "This module called the \"Private.Update Purge Strategy Settings\" private request."
            n287 = event-data() -> ("Purge Settings"=w285:T5)  [unwired: 1 in]
          }
          event User Event {
            # "Another Module called the \"Force Purge\" API Method."
            n288 = event-data() -> ()  [unwired: 1 in, 1 out]
            n289 = call "Force Anode Puge--SubVI.vi"("Anode Request Events"=w287, "error in (no error)"=w289, "Purge Settings in"=w291, "Purge State in"=w294, "Refnum in"=w293) -> ("error out"=w290:errorcluster, "Purge Settings out"=w292:T5, "Purge State out 2"=w295:T31, "Refnum out"=w288:refnum<k21>)  [unwired: 3 in]
          }
        }
        n290 = call-dynamic "Delacor_lib_QMH_Error Handler - Helper Loop.vi"("Error Debug"=w245, "error in"=w247, "Message Queue in"=w246) -> ()  [unwired: 7 in, 2 out]
      }
      n291 = while "DQMH_HELPER_LOOP" {
        shift-right: [w75] -> _
        shift-left: -1 -> [w74]
        shift-right: [w72] -> w35
        shift-left: w34 -> [w73]
        tunnel: w61 -> [w69]
        shift-right: [w66] -> _
        shift-left: _ -> [w67]
        stop <- w71 stop-if-true
        w68 = "H2 Sensor CAN Helper Loop"  # DQMH_HELPER_LOOP_NAME
        # "H2 Sensor CAN Helper Loop"
        n292 = event "DQMH_HELPER_EVENT_STRUCTURE" shown="[0] Timeout" {
          selector: w73 -> [_ _ _ _]
          dyn-events: [_ _ _ _] -> w72
          timeout: w74 -> [_ _ _ _]
          tunnel: w74 -> [w81 _ _ w101]
          tunnel: [w81 1000 -1 w101] -> w75
          tunnel: [_ _ _ TRUE] -> w71
          tunnel: [w76 _ w94 w98] -> w70
          tunnel: w69 -> [_ _ _ _]
          tunnel: w67 -> [w80 w88 w93 w99]
          tunnel: [w79 w91 w93 w99] -> w66
          event Timeout {
            n293 = event-data() -> ()  [unwired: 1 in, 1 out]
            n294 = call "Read H2 Sensor Values.vi"("Refnum in"=w80) -> ("error out"=w76:errorcluster, "Data Map"=w77:map{string, dbl}, "data"=→"H2 Sensor Data":dbl[], "Refnum out"=w79:refnum<k21>)  [unwired: 7 in]
            n295 = case shown="Error .." w76 {
              tunnel: w77 -> [w83 _]
              frame No Error {
                n296 = call "Broadcast H2 Sensor Data.vi"("Data Map"=w83) -> ("error out"=w82:errorcluster)  [unwired: 10 in]
                n297 = call <vilib>:"Clear Errors.vi"("error in (no error)"=w82) -> ()  [unwired: 5 in, 2 out]
              }
              frame Error {
                n298 = Wait (ms)(milliseconds to wait=u32 1000) -> (millisecond timer value=w84:u32)
                n299 = flat-sequence {
                  tunnel: w84 -> [_]
                  frame #0 {
                    n300 = call "Wake H2 Sensor Loop.vi"() -> ()  [unwired: 11 in, 1 out]
                  }
                }
              }
            }
          }
          event User Event {
            w92 = u32 1 items=["Off", "On"] ("Interface:CAN:Termination")
            n301 = event-data() -> ()  [unwired: 1 in, 5 out]
            n302 = call <vilib>:"XNET Clear.vi"("session in"=w88) -> ("error out"=w87:errorcluster)  [unwired: 14 in]
            n303 = call <vilib>:"Clear Errors.vi"("error in (no error)"=w87) -> ("error out"=w86:errorcluster)  [unwired: 5 in, 1 out]
            n304 = property class="XNET Session"(reference=refnum<k21> "Session_H2_Sensor" ("XNET Session"), error in=w86, "Intf.CAN.Term"=w92) -> (reference out=w91:refnum<k21>)  [unwired: 1 out]
          }
          event User Event {
            n305 = event-data() -> ()  [unwired: 1 in, 5 out]
            n306 = disable-structure shown="Enabled" {
              disable-tunnel: w93 -> [w97 _]
              disable-tunnel: [w96 _] -> w94
              frame Disabled {
                n307 = call <vilib>:"XNET Clear.vi"("session in"=w97) -> ("error out"=w96:errorcluster)  [unwired: 14 in]
              }
              frame Enabled {
              }
            }
          }
          event User Event {
            n308 = event-data() -> ()  [unwired: 1 in, 1 out]
            n309 = disable-structure shown="Disabled" {
              disable-tunnel: w99 -> [w103 _]
              disable-tunnel: [w102 _] -> w98
              frame Disabled {
                n310 = call <vilib>:"XNET Clear.vi"("session in"=w103) -> ("error out"=w102:errorcluster)  [unwired: 14 in]
              }
              frame Enabled {
              }
            }
          }
        }
        n311 = call-dynamic "Delacor_lib_QMH_Error Handler - Helper Loop.vi"("Error Debug"=w68, "error in"=w70, "Message Queue in"=w69) -> ()  [unwired: 7 in, 2 out]
      }
      n312 = Unregister For Events(event registration refnum=w49) -> ()  [unwired: 1 in, 1 out]
      n313 = Unregister For Events(event registration refnum=w46) -> ()  [unwired: 1 in, 1 out]
      n314 = Unregister For Events(event registration refnum=w42) -> ()  [unwired: 1 in, 1 out]
      n315 = Unregister For Events(event registration refnum=w35) -> ()  [unwired: 1 in, 1 out]
      n316 = Unregister For Events(event registration refnum=w53) -> ()  [unwired: 1 in, 1 out]
    }
    frame Error {
      # "Synchronize Caller Events.vi will inform Start Module.vi that the module has launched and will let the code calling Start Module.vi register for broadcasts and would permit the caller receive the broadcast that an error occurred at launch time."
      n317 = call-dynamic "Delacor_lib_QMH_Release Message Queue.vi"("Message Queue"=w819) -> ()  [unwired: 10 in, 1 out]
      n318 = call "Synchronize Caller Events.vi"("Singleton Module Admin in"=w824) -> ("error out"=w821:errorcluster)  [unwired: 9 in, 1 out]
      n319 = call "Module Name--constant.vi"() -> ("Module Name"=w827:string)  [unwired: 11 in]
      n320 = Format Into String(format string="An error occurred during initialization. %s is no longer running.", w827) -> (resulting string=w825:string)  [unwired: 2 in, 1 out]
      n321 = Merge Errors(w823, w821) -> (w822:errorcluster)
      n322 = call "Error Reported.vi"("Additional Information"=w825, "Error"=w822) -> ()  [unwired: 9 in, 1 out]
    }
  }
  n323 = Merge Errors(w21, w28) -> (w20:errorcluster)
  n324 = call "Close Module.vi"("error in (no error)"=w20, "Module Admin in"=w29) -> ("error out"=w23:errorcluster, "External Launch"=w18:bool, "Module Admin out"=w22:refnum<class "Delacor_lib_QMH_Module Admin.lvclass">)  [unwired: 7 in]
  n325 = Unregister For Events(event registration refnum=w27, error in=w23) -> (error out=w19:errorcluster)
  "error out" <- w19
  n326 = case "External Launch?" shown="True" w18 {
    tunnel: w19 -> [_ w833]
    tunnel: w16 -> [_ w832]
    tunnel: w8 -> [_ w830]
    frame False {
    }
    frame True {
      n327 = call-dynamic <vilib>:"Close.vi"("Panel In"=w832) -> ("Error Out"=w831:errorcluster)  [unwired: 10 in]
      n328 = call <vilib>:"Close.vi"("error in (no error)"=w831, "Controller in"=w830) -> ("error out"=w829:errorcluster)  [unwired: 9 in]
      n329 = case shown="Error" w833 {
        tunnel: w829 -> [_ _]
        frame No Error {
        }
        frame Error {
          n330 = disable-structure shown="Default" {
            frame condition #0 (active) {
              n331 = invoke class="VI" method="FP.Open"("Activate"=TRUE ("Activate?")) -> ()  [unwired: 4 in, 5 out]
            }
            frame condition #1 {
              # "Don't show panel on error if running inside a built EXE."
            }
          }
        }
      }
    }
  }
  n332 = local write "Module Admin"(w22) -> ()
